vi "CC Create Script.vi"(11 "script name in":string) -> (3 "script name out":string)   [LabVIEW 2024]
uses:
  typedefs/CC cluster Exposure.ctl
  Detector/Detector Class/Detector enum Detector Integration Mode.ctl
  typedefs/CC cluster sidereal rate.ctl
  typedefs/CC Dithering.ctl
  typedefs/CC cluster Offset Dithering.ctl
  typedefs/CC Dithering Offsets.ctl
  typedefs/cc cluster muRA muDEC.ctl
  typedefs/CC cluster Random Dithering.ctl
  Detector/FITS/FITS enum Data Type.ctl
  Telescope/CC cluster Telescope Offsets.ctl
  typedefs/CC cluster Object.ctl
  typedefs/CC cluster RA and DEC.ctl
  typedefs/CC Script Step.ctl
  typedefs/CC enum Script Action.ctl
  Scripts/CC Rd Wr Script Creator Defaults.ctl
  typedefs/CC Dithering Map.ctl
  typedefs/CC enum Dithering Types.ctl
  Detector/FITS/FITS cluster Header Row.ctl
  typedefs/CC cluster Script.ctl
  Subsystems/SS typedef cluster Instrument Command Queue Data.ctl
  Scripts/CC Rd Wr Script Action.ctl
  Focus/Focus cluster MoveFocus Command Parameters.ctl
  typedefs/CC cluster Filter Wheel Parameters.ctl
  typedefs/CC cluster Acquire Parameters.ctl
  typedefs/CC cluster Pause Parameters.ctl
  Filter Wheel/Filter Wheel Object/Filter Wheel.lvclass
  Telescope/PRIME Telescope/PRIME Telescope.lvclass
panel:
  in  "Script Path":path
  in  "Delete":bool
  in  "New Button":bool
  in  "Save As Button":bool
  in  "Script Name":u16(ring) items=["SouthernCross"]
  in  "Save Script":bool
  in  "Close":bool
  in  "Script":i32(listbox)
  in  "Tab Control":T1(tab)
  in  "Units":string
  in  "Open Button":bool
  out "FITS Header Template":path
  in  "Save Header":bool
  in  "Add/Replace":bool
  in  "Comment":string
  in  "Value":string
  in  "Header Field":string(combo)
  in  "FITS Header":i32(listbox)
  in  "Type":T2
  in  "RA and DEC String":cluster{"RA":string, "DEC":string}={"RA"="HH:MM:SS.nnn", "DEC"="DEG:arcmin:arcsec.nn"} caption="RA and DEC"
  in  "Obj Add to Script":bool
  in  "Obj Remove":bool
  in  "Object Name":cluster{"Name":string}
  in  "Sidereal Rate":T3
  in  "Obj Add/Replace":bool
  in  "Objects":i32(listbox)
  in  "Proper Motion":T4
  in  "Offsets":T5
  in  "Exp Add to Script":bool
  in  "Exp Remove":bool
  in  "Exp Add/Replace":bool
  in  "Exposure":T6={"Mode"=enum."CDS", "Integration Time"=1.0, "Name"="", "Images"=1}
  in  "Exposures":i32(listbox)
  in  "Add FW 4":bool
  in  "Add FW 3":bool
  in  "Add FW 2":bool
  in  "Add FW 1":bool
  in  "Filter Wheel 4":i32(listbox)
  in  "Filter Wheel 3":i32(listbox)
  in  "Filter Wheel 2":i32(listbox) caption="OuterWheel"
  in  "Filter Wheel 1":i32(listbox) caption="InnerWheel"
  in  "Name":string
  in  "Dither Add to Script":bool
  in  "Dithering Add/Replace":bool
  in  "Dithering":i32(listbox)
  in  "Dithering Remove":bool
  in  "Dither Select":enum32{"Random", "Offset"}(tab)
  in  "Random Dither":T8={"Count"=1, "Radius"=1.0, "Name"=""}
  in  "Dithering Offset":T9
  in  "Add Image Acq":bool
  in  "Acquire Parameters":T12
  in  "Add Macro":bool
  in  "Script to Call":u16(ring)
  in  "Move Telescope":bool
  in  "RA and DEC String 2":cluster{"RA":string, "DEC":string}={"RA"="HH:MM:SS.nnn", "DEC"="DEG:arcmin:arcsec.nn"} caption="RA and DEC"
  in  "Telescope Focus":T13
  in  "Message for User":string
  in  "Add Ask":bool caption="Add Ask to Script"
  in  "Seconds to Pause":dbl=10.0
  in  "Add Pause":bool caption="Add Pause to Script"
  in  "Home":bool
  in  "Absolute":bool
  in  "Relative":bool
  in  "Steps":i32
  in  "Select Motor (0:n-1)":i32 min=0 max=3 step=1
  in  "Add No-op":bool caption="Add Noop to Script"
  out "Script As Text":string="DefineObject Alpha1234 Standard RA=123.456 DEC=456.789\nDefineExposure Number=1,Groups=1,ReadoutsPerGroup=1,TimeBetweenGroups=10,TimeBetweenReadouts=10\nDefineDithering DEC=0,-10,+10 RA=0,-10,+10\nMoveFilter A,B\nAcquireImages [This command acquires image at every dithering position]\n\n"
  in  "Send":bool
  in  "Script Line":string
  # "Select a Configuration (PRIME or RIMAS, FilterWheel, etc.)"
  # "Add warning for invalid combinationss"
  # "\"\t   Y, J, or H can go with Open or Narrow only\n\"\t  Z must go with Open\n\"\t Dark can go with anything\n\"\t Open can go with anything\n\"\t Narrow can only go with T, J, H"
  # "arcseconds"
  # "arcseconds"
  # "Telescope Pointing"
  # "Focus"
  # "The noop command is used for testing purposes. There are no parameters."
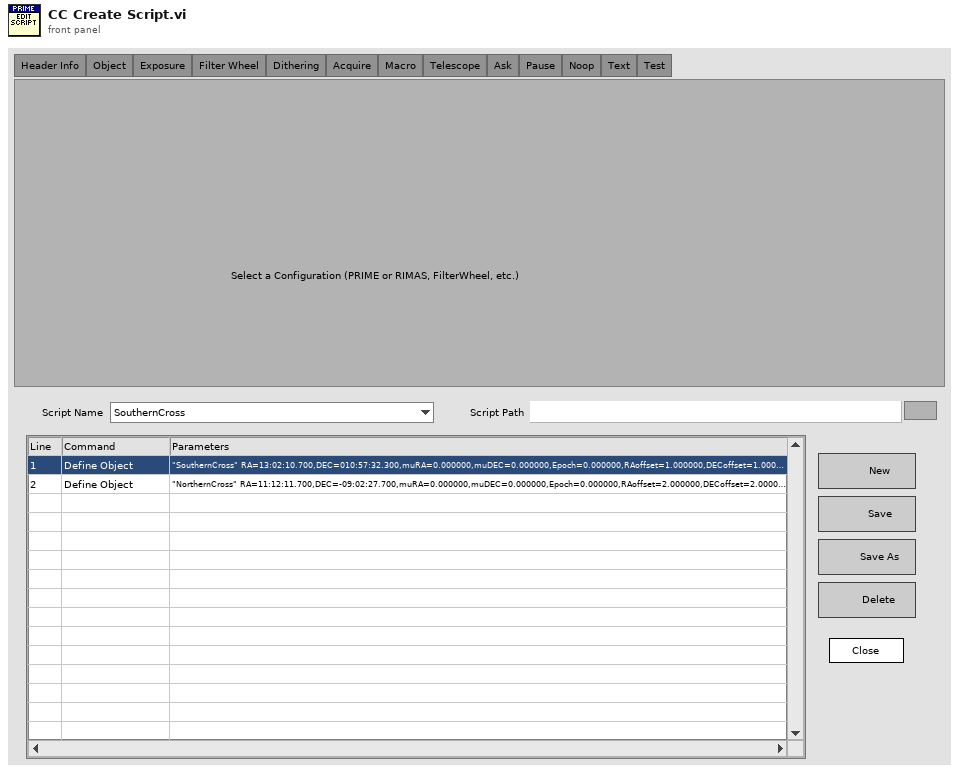
[diagram p1: front panel]
types:
  T1 = enum32{"Setup", "Header Info", "Object", "Exposure", "Filter Wheel", "Dithering", "Acquire", "Macro", "Telescope", "Ask", "Pause", "PicoMotors", "Noop", "Text", "Test"}
  T2 = typedef "FITS enum Data Type.ctl" = enum16{"String", "Integer", "Float"}
  T3 = typedef "CC cluster sidereal rate.ctl" = cluster{"dRA":dbl, "dDEC":dbl}
  T4 = typedef "cc cluster muRA muDEC.ctl" = cluster{"muRA":dbl, "muDEC":dbl, "Epoch":dbl}
  T5 = typedef "CC cluster Telescope Offsets.ctl" = cluster{"RA":dbl, "DEC":dbl, "ROT":dbl}
  T6 = typedef "CC cluster Exposure.ctl" = cluster{"Mode":T7, "Integration Time":dbl, "Name":string, "Images":i32}
  T7 = typedef "Detector enum Detector Integration Mode.ctl" = enum16{"SSR", "CDS", "MEAN", "MEDIAN", "MODE", "MIIN", "MAX"}
  T8 = typedef "CC cluster Random Dithering.ctl" = cluster{"Count":i32, "Radius":dbl, "Name":string}
  T9 = typedef "CC Dithering.ctl" = cluster{"Name":string, "Dithering Offsets":T10}
  T10 = typedef "CC cluster Offset Dithering.ctl" = cluster{"Offsets":T11[]}
  T11 = typedef "CC Dithering Offsets.ctl" = cluster{"DEC":dbl, "RA":dbl}
  T12 = cluster{"Object":string, "Exposure":string, "Dithering":string}
  T13 = cluster{"Focus Home":bool, "Move Focus":bool, "Position":dbl}
  T14 = typedef "CC cluster Object.ctl" = cluster{"Object":cluster{"Name":string}, "Sidereal Rate":T3, "RA and DEC":T15, "muRA muDEC Epoch":T4, "Offsets":T5}
  T15 = typedef "CC cluster RA and DEC.ctl" = cluster{"RA":dbl, "DEC":dbl}
  T16 = typedef "CC Script Step.ctl" = cluster{"Action":T17, "Data":variant}
  T17 = typedef "CC enum Script Action.ctl" = enum16{"Noop", "Define Object", "Define Exposure", "Define Dithering", "Acquire Images", "Set Filter Wheel", "Telescope Home", "Telescope Move", "Telescope RA DEC", "Focus Move Relative", "Focus Move Absolute", "Focus Set Home", "Macro", "Pause", "Ask User", "Define Random Dither"}
  T18 = typedef "CC Rd Wr Script Creator Defaults.ctl" = cluster{"Script":string, "Script Path":path}
  T19 = typedef "CC Dithering Map.ctl" = cluster{"Name":string, "Dithering Offsets":T9, "Dithering Type":T20, "Random Dither":T8}
  T20 = typedef "CC enum Dithering Types.ctl" = enum16{"Random", "Offsets", "None"}
  T21 = typedef "FITS cluster Header Row.ctl" = cluster{"Field Name":string, "Type":T2, "Value":string, "Comment":string, "Units":string}
  T22 = cluster{"state":refnum<user-event>, "Object Map":map{string, T14}, "curr object":string, "Exp Map":map{string, T6}, "Script":T16[], "Settings":T18, "test":T16[], "Dither Map":map{string, T19}, "Hdr Map":map{string, T21}}
  T23 = typedef "CC cluster Script.ctl" = cluster{"Name":string, "Script":T16[]}
  T24 = typedef "CC Rd Wr Script Action.ctl" = enum16{"Read", "Write", "List", "Delete"}
  T25 = typedef "SS typedef cluster Instrument Command Queue Data.ctl" = cluster{"Cmd":string, "Parameters":variant}
  T26 = typedef "Focus cluster MoveFocus Command Parameters.ctl" = cluster{"Motor":i32, "Position":i32}
  T27 = typedef "CC cluster Filter Wheel Parameters.ctl" = cluster{"Wheel":i32, "Filter":i32}
  T28 = enum32{"Setup", "Object", "Exposure", "Dithering", "Acquire", "Filter Wheel", "Focus", "Macro", "Ask", "Pause", "Noop", "Text", "Test"}
  T29 = enum32{"Setup", "Object", "Exposure", "Dithering", "Acquire", "Filter Wheel", "Focus", "Ask", "Pause", "Noop", "Text", "Test"}
  T30 = typedef "CC cluster Acquire Parameters.ctl" = cluster{"Object":string, "Exposure":string, "Dithering":string}
  T31 = enum32{"Setup", "Object", "Exposure", "Filter Wheel", "Dithering", "Acquire", "Macro", "Telescope", "Ask", "Pause", "PicoMotors", "Noop", "Text", "Test"}
  T32 = typedef "CC cluster Pause Parameters.ctl" = cluster{"Time (s)":dbl}
  T33 = typedef "CC cluster Script Panel Defaults.ctl" = cluster{"Script Name":string, "Script Path":path}
  T34 = typedef "RIMAS Detector Config.ctl" = cluster{"Detector":u16, "Offsets":u16[][], "Detector Computer":T35, "FITS hdr template0":path, "FITS hdr template1":path, "FITS Data File Path":path, "FITS Detector Settings":T36, "Sim Folder":path, "Integration Mode":T7, "Integration Time":dbl, "Frame Int Time":dbl}
  T35 = typedef "RIMAS Detector Server Config.ctl" = cluster{"Machine":string, "Password":string, "FITS File Path":string, "Port":u16, "Header Path":string, "Name":string}
  T36 = typedef "RIMAS Observation Config.ctl" = cluster{"Exp Time Short":dbl, "# of Frames":dbl, "Exp Time Long":dbl, "# of Groups":dbl, "Object Name":string, "Object":string, "Obs Type":string, "Image Type":string, "Observer":string, "Observer Affiliation":string}
  T37 = typedef "CC cluster Hardware Config.ctl" = cluster{"Installed Hardware":T38[]}
  T38 = typedef "CC cluster Device Index.ctl" = cluster{"Device Type Name":string, "Curr Device Name":string, "All Instances":string[]}
  T39 = typedef "Filter Wheel.lvclass/Filter Wheel configuration.ctl" = cluster{"Num Wheels":i32, "Filters":T40[], "Invalid Combinations":i32[][], "Addr":refnum<visa-resource-name>, "Name":string, "Simulate":bool, "Homing Parameters":T41, "Default Speed":u16}
  T40 = typedef "Filter Wheel.lvclass/Filter Wheel Details.ctl" = cluster{"Names":string[], "Relative Position":i32[], "Wheel Name":string}
  T41 = typedef "Filter Wheel Arduino Homing cluster.ctl" = cluster{"Direction (F: CW)":bool, "Speed":i32, "Accel":i32, "Min Distance":i32, "Short Leg":i32, "Error Cnts":i32}
  T42 = typedef "LVPoint32TypeDef.ctl" = cluster{"Horizontal":i32, "Vertical":i32}
  T43 = typedef "LVRowAndColumnTypeDef.ctl" = cluster{"Row":i32, "Column":i32}
  T44 = enum32{"Setup", "Object", "Exposure", "Dithering", "Acquire", "Filter Wheel", "Ask", "Pause", "Noop", "Text"}
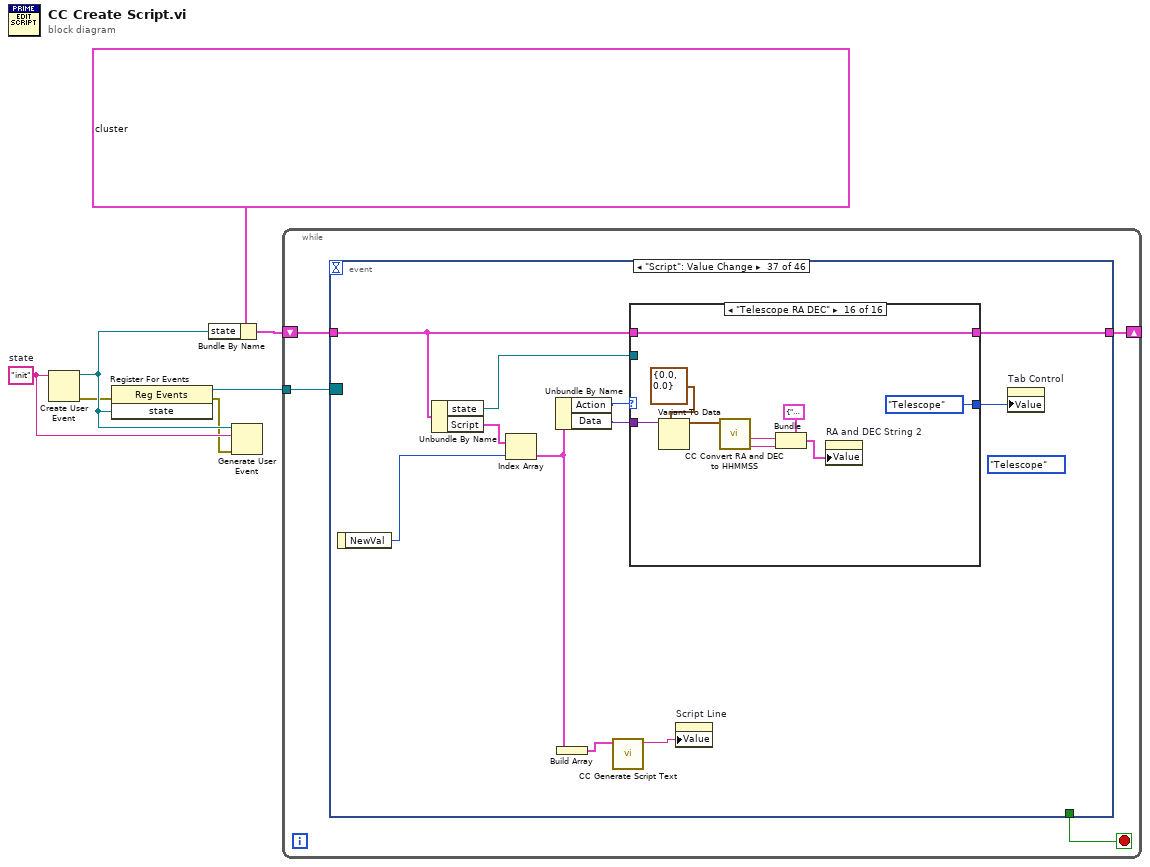
[diagram p0: block diagram]
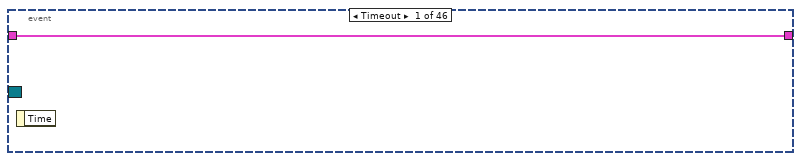
[diagram p2: hidden frame]
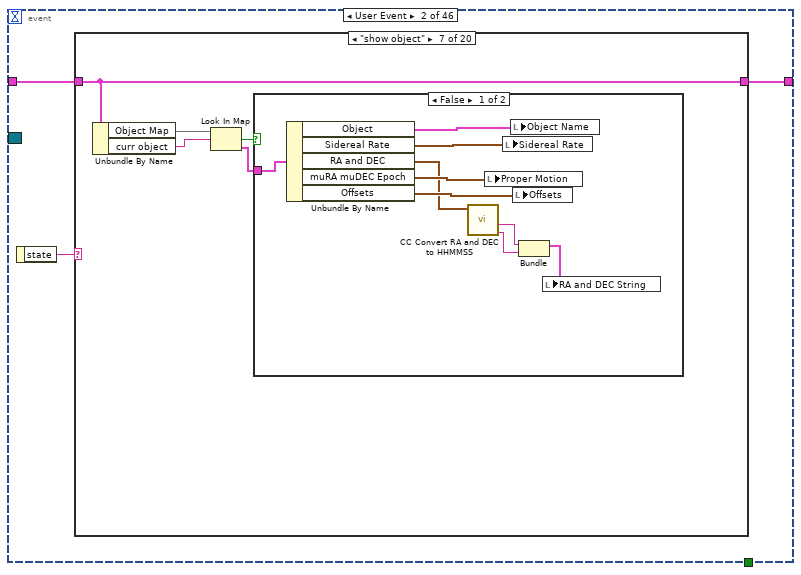
[diagram p3: hidden frame]
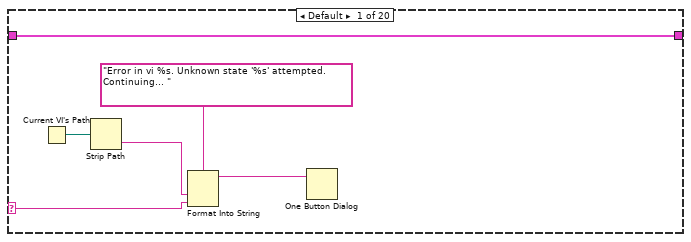
[diagram p4: hidden frame]
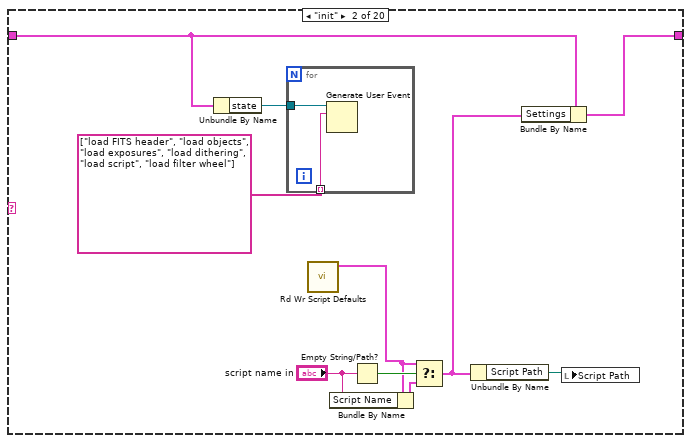
[diagram p5: hidden frame]
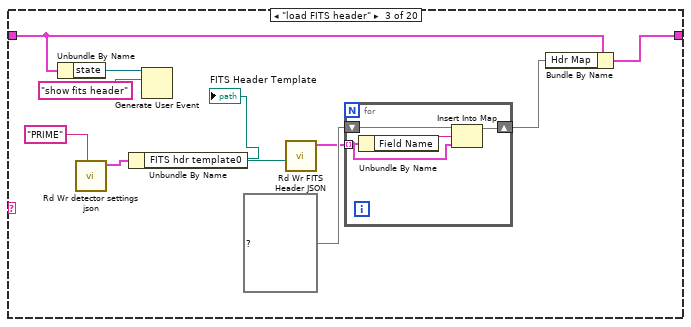
[diagram p6: hidden frame]
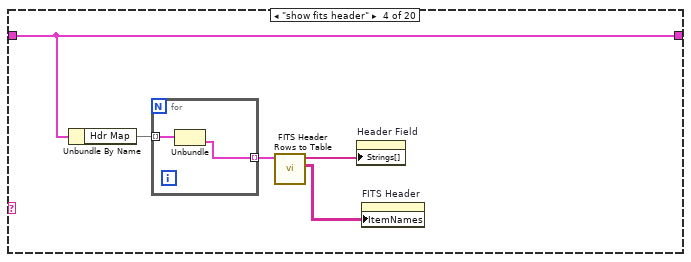
[diagram p7: hidden frame]
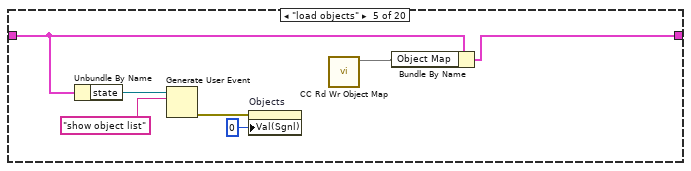
[diagram p8: hidden frame]
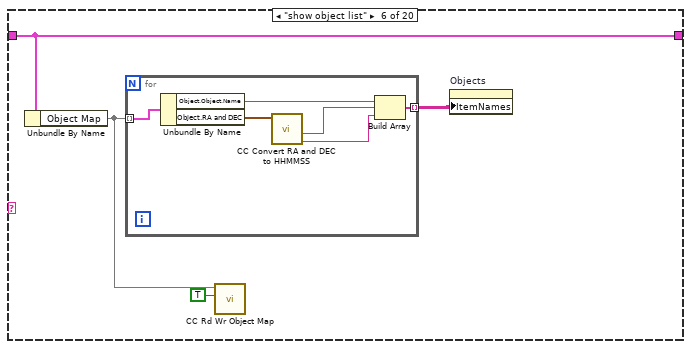
[diagram p9: hidden frame]
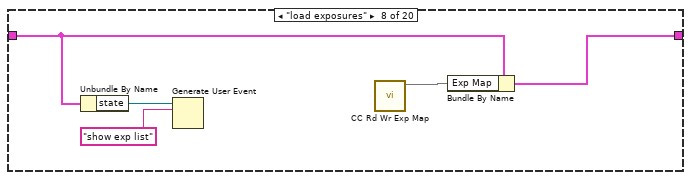
[diagram p11: hidden frame]
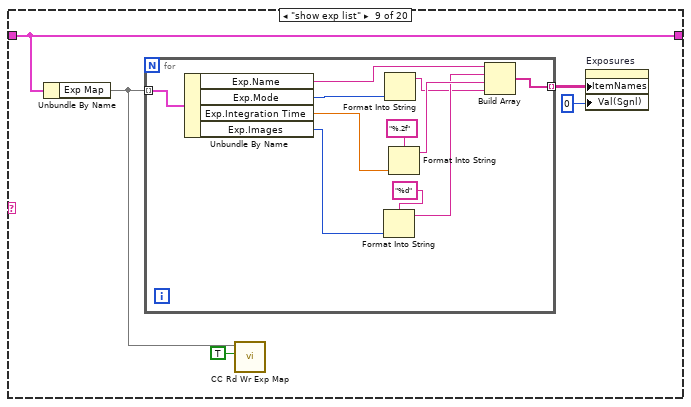
[diagram p12: hidden frame]
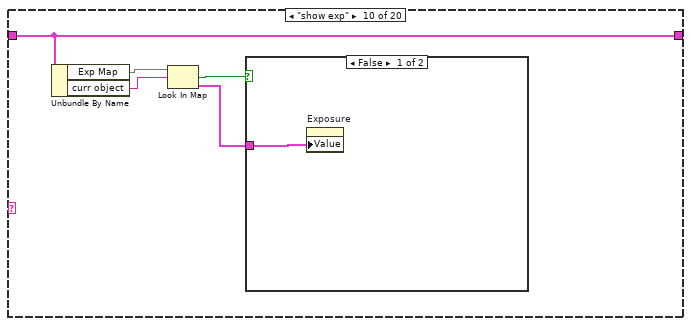
[diagram p13: hidden frame]
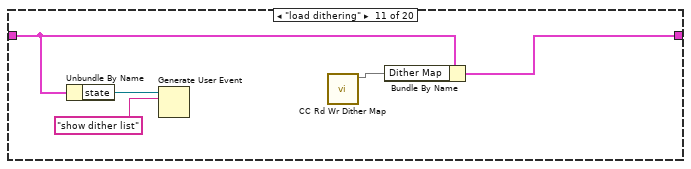
[diagram p15: hidden frame]
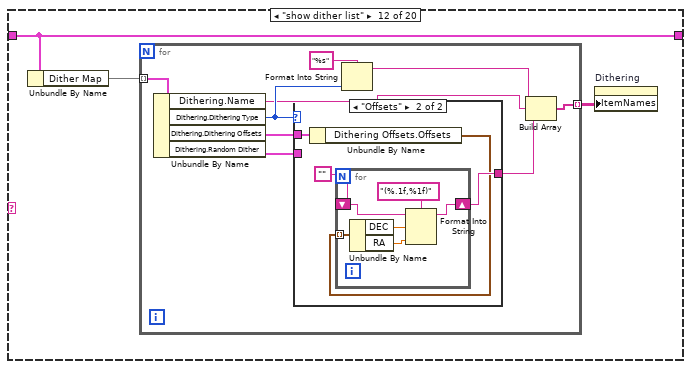
[diagram p16: hidden frame]
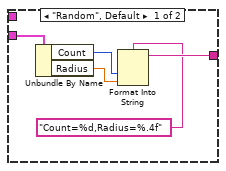
[diagram p17: hidden frame]
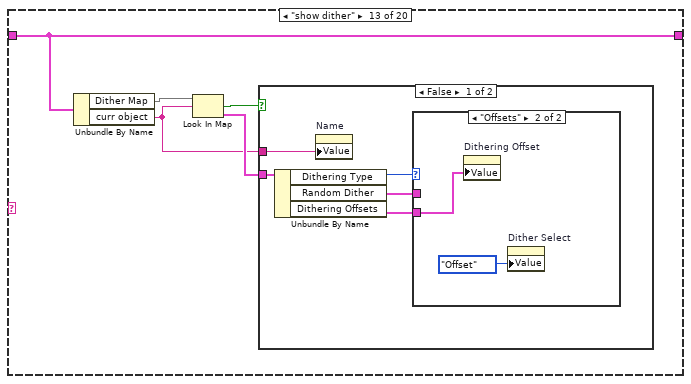
[diagram p18: hidden frame]
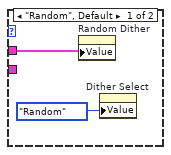
[diagram p19: hidden frame]
diagram:
  w3 = "init"  # state
  n1 = Create User Event(user event datatype=w3) -> (user event=w5:refnum<user-event>, error out=w1:errorcluster)  [unwired: 1 in]
  n2 = register-events(error in=w1, w5) -> (reference out=w4:refnum<event-registration>, error out=w2:errorcluster)  [unwired: 1 in]
  n3 = Bundle By Name(cluster=T22 {"state"=refnum, "Object Map"={}, "curr object"="", "Exp Map"={}, "Script"=[], "Settings"={"Script"="", "Script Path"=path ""}, "test"=[], "Dither Map"={}, "Hdr Map"={}}, "state"=w5) -> (w6:T22)
  n4 = Generate User Event(user event=w5, event data cluster=w3, error in=w2) -> ()  [unwired: 1 in, 2 out]
  n5 = while {
    tunnel: w4 -> [w11]
    shift-right: [w9] -> _
    shift-left: w6 -> [w10]
    stop <- w8 stop-if-true
    n6 = event shown="[36] \"Script\": Value Change" {
      selector: w11 -> [_ _ _ _ _ _ _ _ _ _ _ _ _ _ _ _ _ _ _ _ _ _ _ _ _ _ _ _ _ _ _ _ _ _ _ _ _ _ _ _ _ _ _ _ _ _]
      dyn-events: _ -> [_ _ _ _ _ _ _ _ _ _ _ _ _ _ _ _ _ _ _ _ _ _ _ _ _ _ _ _ _ _ _ _ _ _ _ _ _ _ _ _ _ _ _ _ _ _]
      timeout: _ -> [_ _ _ _ _ _ _ _ _ _ _ _ _ _ _ _ _ _ _ _ _ _ _ _ _ _ _ _ _ _ _ _ _ _ _ _ _ _ _ _ _ _ _ _ _ _]
      tunnel: w10 -> [w12 w14 w271 w283 w285 w288 w310 w324 w328 w339 w341 w352 w365 w386 w390 w402 w412 w432 w447 w470 w495 w526 w537 w543 w558 w572 w609 w615 w636 w675 w686 w698 w703 w714 w720 w728 w779 w886 w900 w913 w922 w934 w949 w951 w985 w989]
      tunnel: [w12 w13 w272 w283 w285 w289 w310 w324 w328 w336 w342 w353 w366 w387 w391 w403 w413 w433 w446 w469 w494 w527 w538 w544 w559 w573 w610 w614 w636 w676 w687 w698 w702 w714 w721 w728 w778 w887 w901 w914 w923 w935 w949 w950 w985 w989] -> w9
      tunnel: [_ _ _ _ _ _ _ _ _ _ _ _ _ _ _ _ _ _ _ _ _ _ _ _ _ _ _ _ _ _ _ _ _ _ _ _ _ _ _ _ _ _ _ _ _ "Close"] -> w8
      event Timeout {
        n7 = event-data() -> ()  [unwired: 1 in, 1 out]
      }
      event User Event {
        n8 = event-data() -> ("state"=w15:string)  [unwired: 1 in]
        n9 = case shown="\"show object\"" w15 {
          selector: w15 -> [w20 _ _ _ _ _ _ _ _ _ _ _ _ _ _ _ _ _ _ _]
          tunnel: w14 -> [w16 w28 w36 w50 w59 w64 w76 w86 w95 w111 w114 w120 w146 w163 w202 w230 w235 w250 w255 w258]
          tunnel: [w16 w29 w41 w50 w61 w64 w76 w89 w95 w111 w117 w120 w146 w164 w202 w230 w235 w250 w255 w258] -> w13
          frame Default {
            n10 = Current VI's Path() -> (path=w19:path)
            n11 = Strip Path(path=w19) -> (name=w18:string)  [unwired: 1 out]
            n12 = Format Into String(format string="Error in vi %s. Unknown state '%s' attempted. Continuing... ", w18, w20) -> (resulting string=w17:string)  [unwired: 2 in, 1 out]
            n13 = One Button Dialog(message=w17) -> ()  [unwired: 1 in, 1 out]
          }
          frame "init" {
            n14 = Unbundle By Name(w28) -> ("state"=w31:refnum<user-event>)
            n15 = for {
              tunnel: w31 -> [w33]
              tunnel: string[] ["load FITS header", "load objects", "load exposures", "load dithering", "load script", "load filter wheel"] -> [w32] mode=indexing
              n16 = Generate User Event(user event=w33, event data cluster=w32) -> ()  [unwired: 2 in, 2 out]
            }
            n17 = call "Rd Wr Script Defaults.vi"() -> ("Script Settings"=w22:T33)  [unwired: 10 in, 1 out]
            n18 = Bundle By Name(cluster=w22, "Script Name"="script name in") -> (w25:T33)
            n19 = Empty String/Path?(string/path="script name in") -> (empty?=w27:bool)
            n20 = Select(t=w22, s=w27, f=w25) -> (s? t:f=w23:T33)
            n21 = Unbundle By Name(w23) -> ("Script Path"=w24:path)
            n22 = Bundle By Name(cluster=w28, "Settings"=w23) -> (w29:T22)
            n23 = local write "Script Path"(w24) -> ()
          }
          frame "load FITS header" {
            n24 = Unbundle By Name(w36) -> ("state"=w35:refnum<user-event>)
            n25 = call "Rd Wr detector settings json.vi"("Detector Name"="PRIME") -> ("Detector Config"=w42:T34)  [unwired: 9 in, 1 out]
            n26 = Unbundle By Name(w42) -> ("FITS hdr template0"=w40:path)
            "FITS Header Template" <- w40
            n27 = Generate User Event(user event=w35, event data cluster="show fits header" ("event data")) -> ()  [unwired: 2 in, 2 out]
            n28 = call "Rd Wr FITS Header JSON.vi"("FITS Template"=w40) -> ("FITS Hdr Rows"=w37:T21[])  [unwired: 9 in, 1 out]
            n29 = for {
              tunnel: w37 -> [w45] mode=indexing
              shift-right: [w44] -> w38
              shift-left: map{string, T21} {} ("Hdr Map") -> [w47]
              n30 = Unbundle By Name(w45) -> ("Field Name"=w46:string)
              n31 = Insert Into Map(map in=w47, key=w46, value=w45) -> (map out=w44:map{string, T21})  [unwired: 2 out]
            }
            n32 = Bundle By Name(cluster=w36, "Hdr Map"=w38) -> (w41:T22)
          }
          frame "show fits header" {
            n33 = Unbundle By Name(w50) -> ("Hdr Map"=w49:map{string, T21})
            n34 = for {
              tunnel: w49 -> [w54] mode=indexing
              tunnel: [w53] -> w48 mode=indexing
              n35 = Unbundle(w54) -> (w53:T21)  [unwired: 1 out]
            }
            n36 = call "FITS Header Rows to Table.vi"("FITS Hdr Rows"=w48) -> ("table"=w51:string[][], "Keywords"=w52:string[])  [unwired: 9 in]
            n37 = property on="Header Field" class="CmbBox"("Strings[]"=w52) -> ()  [unwired: 2 in, 2 out]
            n38 = property on="FITS Header" class="MCListbox (strict)"("ItemNames"=w51) -> ()  [unwired: 2 in, 2 out]
          }
          frame "load objects" {
            n39 = Unbundle By Name(w59) -> ("state"=w58:refnum<user-event>)
            n40 = Generate User Event(user event=w58, event data cluster="show object list" ("event data")) -> (error out=w56:errorcluster)  [unwired: 2 in, 1 out]
            n41 = property on="Objects" class="MCListbox (strict)"(error in=w56, "Val(Sgnl)"=0 ("Value (Signaling)")) -> ()  [unwired: 1 in, 2 out]
            n42 = call "CC Rd Wr Object Map.vi"() -> ("Object Map in"=w60:map{string, T14})  [unwired: 10 in, 1 out]
            n43 = Bundle By Name(cluster=w59, "Object Map"=w60) -> (w61:T22)
          }
          frame "show object list" {
            n44 = Unbundle By Name(w64) -> ("Object Map"=w63:map{string, T14})
            n45 = for {
              tunnel: w63 -> [w71] mode=indexing
              tunnel: [w69] -> w65 mode=indexing
              n46 = Unbundle By Name(w71) -> ("Object.Object.Name"=w70:string, "Object.RA and DEC"=w68:T15)
              n47 = call "CC Convert RA and DEC to HHMMSS.vi"("RA and DEC"=w68) -> ("DEC String"=w66:string, "RA String"=w67:string)  [unwired: 9 in]
              n48 = Build Array(w70, w67, w66) -> (w69:string[])
            }
            n49 = call "CC Rd Wr Object Map.vi"("Write? (F:Read)"=TRUE, "Object Map in"=w63) -> ()  [unwired: 8 in, 2 out]
            n50 = property on="Objects" class="MCListbox (strict)"("ItemNames"=w65) -> ()  [unwired: 2 in, 2 out]
          }
          frame "show object" {
            n51 = Unbundle By Name(w76) -> ("Object Map"=w75:map{string, T14}, "curr object"=w74:string)
            n52 = Look In Map(map=w75, key=w74) -> (key not found?=w73:bool, value=w72:T14)  [unwired: 1 in]
            n53 = case shown="False" w73 {
              tunnel: w72 -> [w85 _]
              frame False {
                n54 = Unbundle By Name(w85) -> ("Object"=w84:cluster{"Name":string}, "Sidereal Rate"=w83:T3, "RA and DEC"=w80:T15, "muRA muDEC Epoch"=w82:T4, "Offsets"=w81:T5)
                n55 = call "CC Convert RA and DEC to HHMMSS.vi"("RA and DEC"=w80) -> ("DEC String"=w78:string, "RA String"=w79:string)  [unwired: 9 in]
                n56 = local write "Proper Motion"(w82) -> ()
                n57 = local write "Sidereal Rate"(w83) -> ()
                n58 = local write "Object Name"(w84) -> ()
                n59 = local write "Offsets"(w81) -> ()
                n60 = Bundle("RA String"=w79, "DEC String"=w78) -> (w77:cluster{"RA String":string, "DEC String":string})  [unwired: 1 in]
                n61 = local write "RA and DEC String"(w77) -> ()
              }
              frame True {
              }
            }
          }
          frame "load exposures" {
            n62 = Unbundle By Name(w86) -> ("state"=w88:refnum<user-event>)
            n63 = Generate User Event(user event=w88, event data cluster="show exp list" ("event data")) -> ()  [unwired: 2 in, 2 out]
            n64 = call "CC Rd Wr Exp Map.vi"() -> ("Exp Map"=w90:map{string, T6})  [unwired: 10 in, 1 out]
            n65 = Bundle By Name(cluster=w86, "Exp Map"=w90) -> (w89:T22)
          }
          frame "show exp list" {
            n66 = Unbundle By Name(w95) -> ("Exp Map"=w93:map{string, T6})
            n67 = for {
              tunnel: w93 -> [w106] mode=indexing
              tunnel: [w102] -> w94 mode=indexing
              n68 = Unbundle By Name(w106) -> ("Exp.Name"=w105:string, "Exp.Mode"=w104:T7, "Exp.Integration Time"=w101:dbl, "Exp.Images"=w99:i32)
              n69 = Format Into String(format string="%d", w99) -> (resulting string=w97:string)  [unwired: 2 in, 1 out]
              n70 = Format Into String(w104) -> (resulting string=w96:string)  [unwired: 3 in, 1 out]
              n71 = Format Into String(format string="%.2f", w101) -> (resulting string=w100:string)  [unwired: 2 in, 1 out]
              n72 = Build Array(w105, w97, w100, w96) -> (w102:string[])
            }
            n73 = call "CC Rd Wr Exp Map.vi"("Write? (F:Read)"=TRUE, "Exp Map"=w93) -> ()  [unwired: 8 in, 2 out]
            n74 = property on="Exposures" class="MCListbox (strict)"("ItemNames"=w94, "Val(Sgnl)"=0 ("Value (Signaling)")) -> ()  [unwired: 2 in, 2 out]
          }
          frame "show exp" {
            n75 = Unbundle By Name(w111) -> ("Exp Map"=w110:map{string, T6}, "curr object"=w109:string)
            n76 = Look In Map(map=w110, key=w109) -> (key not found?=w108:bool, value=w107:T6)  [unwired: 1 in]
            n77 = case shown="False" w108 {
              tunnel: w107 -> [w112 _]
              frame False {
                n78 = property on="Exposure" class="Clust (strict)"("Value"=w112) -> ()  [unwired: 2 in, 2 out]
              }
              frame True {
              }
            }
          }
          frame "load dithering" {
            n79 = Unbundle By Name(w114) -> ("state"=w116:refnum<user-event>)
            n80 = Generate User Event(user event=w116, event data cluster="show dither list" ("event data")) -> ()  [unwired: 2 in, 2 out]
            n81 = call "CC Rd Wr Dither Map.vi"() -> ("Dither Map"=w113:map{string, T19})  [unwired: 10 in, 1 out]
            n82 = Bundle By Name(cluster=w114, "Dither Map"=w113) -> (w117:T22)
          }
          frame "show dither list" {
            n83 = Unbundle By Name(w120) -> ("Dither Map"=w118:map{string, T19})
            n84 = for {
              tunnel: w118 -> [w129] mode=indexing
              tunnel: [w126] -> w119 mode=indexing
              n85 = Unbundle By Name(w129) -> ("Dithering.Name"=w121:string, "Dithering.Dithering Type"=w123:T20, "Dithering.Dithering Offsets"=w128:T9, "Dithering.Random Dither"=w122:T8)
              n86 = case shown="\"Offsets\"" w123 {
                tunnel: w128 -> [_ w136]
                tunnel: [w131 w137] -> w127
                tunnel: w122 -> [w134 _]
                frame "Random", Default {
                  n87 = Unbundle By Name(w134) -> ("Count"=w133:i32, "Radius"=w132:dbl)
                  n88 = Format Into String(format string="Count=%d,Radius=%.4f", w133, w132) -> (resulting string=w131:string)  [unwired: 2 in, 1 out]
                }
                frame "Offsets" {
                  n89 = Unbundle By Name(w136) -> ("Dithering Offsets.Offsets"=w135:T11[])
                  n90 = for {
                    tunnel: w135 -> [w143] mode=indexing
                    shift-right: [w139] -> w137
                    shift-left: "" -> [w140]
                    n91 = Unbundle By Name(w143) -> ("DEC"=w142:dbl, "RA"=w141:dbl)
                    n92 = Format Into String(format string="(%.1f,%1f)", initial string=w140, w142, w141) -> (resulting string=w139:string)  [unwired: 1 in, 1 out]
                  }
                }
              }
              n93 = Format Into String(format string="%s", w123) -> (resulting string=w124:string)  [unwired: 2 in, 1 out]
              n94 = Build Array(w124, w121, w127) -> (w126:string[])
            }
            n95 = property on="Dithering" class="MCListbox (strict)"("ItemNames"=w119) -> ()  [unwired: 2 in, 2 out]
          }
          frame "show dither" {
            n96 = Unbundle By Name(w146) -> ("Dither Map"=w149:map{string, T19}, "curr object"=w145:string)
            n97 = Look In Map(map=w149, key=w145) -> (key not found?=w148:bool, value=w147:T19)  [unwired: 1 in]
            n98 = case shown="False" w148 {
              tunnel: w147 -> [w154 _]
              tunnel: w145 -> [w150 _]
              frame False {
                n99 = Unbundle By Name(w154) -> ("Dithering Type"=w153:T20, "Random Dither"=w151:T8, "Dithering Offsets"=w152:T9)
                n100 = property on="Name" class="Str"("Value"=w150) -> ()  [unwired: 2 in, 2 out]
                n101 = case shown="\"Offsets\"" w153 {
                  tunnel: w152 -> [_ w158]
                  tunnel: w151 -> [w156 _]
                  frame "Random", Default {
                    n102 = property on="Random Dither" class="Clust (strict)"("Value"=w156) -> ()  [unwired: 2 in, 2 out]
                    n103 = property on="Dither Select" class="TabCtl (strict)"("Value"=enum32{"Random", "Offset"}."Random" ("Dither Select")) -> ()  [unwired: 2 in, 2 out]
                  }
                  frame "Offsets" {
                    n104 = property on="Dithering Offset" class="Clust (strict)"("Value"=w158) -> ()  [unwired: 2 in, 2 out]
                    n105 = property on="Dither Select" class="TabCtl (strict)"("Value"=enum32{"Random", "Offset"}."Offset" ("Dither Select")) -> ()  [unwired: 2 in, 2 out]
                  }
                }
              }
              frame True {
              }
            }
          }
          frame "load script" {
            n106 = Unbundle By Name(w163) -> ("Settings.Script"=w161:string, "Settings.Script Path"=w159:path, "state"=w162:refnum<user-event>)
            n107 = Empty String/Path?(string/path=w161) -> (empty?=w160:bool)
            n108 = case shown="True" w160 {
              tunnel: [w175 w182] -> w164
              tunnel: w163 -> [w174 w182]
              tunnel: w162 -> [w173 _]
              tunnel: w161 -> [w169 _]
              tunnel: w159 -> [w165 _]
              frame False {
                n109 = Bundle By Name(cluster=T23 {"Name"="", "Script"=[]} ("Script"), "Name"=w169) -> (w178:T23)
                n110 = Generate User Event(user event=w173, event data cluster="show script" ("event data")) -> ()  [unwired: 2 in, 2 out]
                n111 = call "CC Rd Wr Script.vi"("Script Path"=w165, "Script"=w178) -> ("Syntax Errors"=w170:string, "Script List"=w168:string[], "Script"=w177:T23, "Script Ok?"=w171:bool)  [unwired: 4 in, 2 out]
                n112 = Unbundle By Name(w177) -> ("Script"=w176:T16[])
                n113 = Search 1D Array(1D array=w168, element=w169) -> (index of element=w167:i32)  [unwired: 1 in]
                n114 = case shown="False" w171 {
                  tunnel: w170 -> [w180 _]
                  frame False {
                    n115 = One Button Dialog(message=w180) -> ()  [unwired: 1 in, 1 out]
                  }
                  frame True {
                  }
                }
                n116 = property on="Script Name" class="Ring (strict)"("Strings []"=w168, "Value"=w167) -> ()  [unwired: 2 in, 2 out]
                n117 = Bundle By Name(cluster=w174, "Script"=w176) -> (w175:T22)
                n118 = Delete From Array(array=w168, index=w167) -> (array with subset deleted=w166:string[])  [unwired: 1 in, 1 out]
                n119 = property on="Script to Call" class="Ring (strict)"("Strings []"=w166) -> ()  [unwired: 2 in, 2 out]
              }
              frame True {
                n120 = property on="Script" class="MCListbox (strict)"("ItemNames"=string[][] [] ("Item Names")) -> ()  [unwired: 2 in, 2 out]
              }
            }
          }
          frame "load filter wheel" {
            n121 = call "CC Rd Wr Hardware Configuration.vi"() -> ("Hardware Config out"=w185:T37)  [unwired: 9 in, 2 out]
            n122 = control-ref of="Filter Wheel 4"() -> (w197:refnum<vi>)
            n123 = control-ref of="Add FW 1"() -> (w192:refnum<vi>)
            n124 = control-ref of="Add FW 2"() -> (w189:refnum<vi>)
            n125 = control-ref of="Add FW 3"() -> (w190:refnum<vi>)
            n126 = control-ref of="Add FW 4"() -> (w191:refnum<vi>)
            n127 = control-ref of="Filter Wheel 3"() -> (w198:refnum<vi>)
            n128 = control-ref of="Filter Wheel 2"() -> (w199:refnum<vi>)
            n129 = control-ref of="Filter Wheel 1"() -> (w200:refnum<vi>)
            n130 = Unbundle By Name(w185) -> ("Installed Hardware"=w184:T38[])
            n131 = Build Array(w192, w189, w190, w191) -> (w188:refnum<vi>[])
            n132 = Build Array(w200, w199, w198, w197) -> (w193:refnum<vi>[])
            n133 = call "CC Get Current Device.vi"("Device Type Name"="filter wheel", "Hardware.Installed Hardware"=w184) -> ("Curr Device Name"=w183:string)  [unwired: 7 in, 2 out]
            n134 = for {
              tunnel: [w208] -> w194 mode=indexing
              tunnel: w193 -> [w207] mode=indexing
              tunnel: w188 -> [w205] mode=indexing
              tunnel: [w203] -> w187 mode=indexing
              n135 = property class="LstBox (strict)"(reference=w207, "Visible"=FALSE) -> (reference out=w208:refnum<vi>)  [unwired: 1 in, 1 out]
              n136 = property class="Bool"(reference=w205, "Visible"=FALSE) -> (reference out=w203:refnum<vi>)  [unwired: 1 in, 1 out]
            }
            n137 = call "Rd Wr Filter Wheel Settings.vi"("Wheel Name"=w183) -> ("Filter Wheel Settings"=w201:T39)  [unwired: 9 in, 1 out]
            n138 = Unbundle By Name(w201) -> ("Filters"=w195:T40[])  [unwired: 1 out]
            n139 = for {
              N: 4 -> [_]
              tunnel: w195 -> [w214] mode=indexing
              tunnel: w194 -> [w213] mode=indexing
              tunnel: w187 -> [w211] mode=indexing
              w210 = TRUE ("Visible")
              n140 = Unbundle By Name(w214) -> ("Names"=w212:string[], "Wheel Name"=w209:string)
              n141 = property class="LstBox (strict)"(reference=w213, "Item Names"=w212, "Visible"=w210, "Caption.Text"=w209) -> ()  [unwired: 1 in, 2 out]
              n142 = property class="Bool"(reference=w211, "Visible"=w210) -> ()  [unwired: 1 in, 2 out]
            }
          }
          frame "save script" {
            n143 = Unbundle By Name(w230) -> ("Settings.Script"=w218:string, "Script"=w231:T16[], "Settings.Script Path"=w215:path)
            n144 = Bundle By Name(cluster=T23 {"Name"="", "Script"=[]} ("Script"), "Name"=w218, "Script"=w231) -> (w232:T23)
            n145 = Obtain Queue(name (unnamed)="Script Queue", element data type=T25 {"Cmd"="", "Parameters"=variant}) -> (queue out=w227:refnum<queue>)  [unwired: 3 in, 2 out]
            n146 = call "CC Rd Wr Script.vi"("Script Path"=w215, "Action"=CC_Rd_Wr_Script_Action."Write", "Script"=w232) -> ("error out"=w220:errorcluster, "Script List"=w219:string[])  [unwired: 3 in, 4 out]
            n147 = Bundle By Name(cluster=T25 {"Cmd"="", "Parameters"=variant} ("element"), "Cmd"="set script", "Parameters"=w218) -> (w223:T25)
            n148 = Search 1D Array(1D array=w219, element=w218) -> (index of element=w217:i32)  [unwired: 1 in]
            n149 = property on="Script Name" class="Ring (strict)"(error in=w220, "Strings []"=w219, "Value"=w217) -> (error out=w224:errorcluster)  [unwired: 1 in, 1 out]
            n150 = Enqueue Element(queue=w227, element=w223, error in (no error)=w224) -> (queue out=w221:refnum<queue>, error out=w222:errorcluster)  [unwired: 1 in, 1 out]
            n151 = Release Queue(queue=w221, error in (no error)=w222) -> ()  [unwired: 1 in, 3 out]
          }
          frame "delete script" {
            n152 = Unbundle By Name(w235) -> ("Settings.Script Path"=w234:path)
            n153 = property on="Script Name" class="Ring (strict)"() -> ("Strings []"=w243:string[], "Value"=w240:u16)  [unwired: 2 in, 2 out]
            n154 = Index Array(array=w243, index=w240) -> (element=w241:string)
            n155 = Bundle By Name(cluster=T23 {"Name"="", "Script"=[]} ("Script"), "Name"=w241) -> (w245:T23)
            n156 = call "CC Rd Wr Script.vi"("Script Path"=w234, "Action"=CC_Rd_Wr_Script_Action."Delete", "Script"=w245) -> ("error out"=w244:errorcluster, "Script List"=w237:string[])  [unwired: 3 in, 4 out]
            n157 = Array Size(array=w237) -> (size(s)=w236:i32)
            n158 = In Range and Coerce(upper limit=w236, x=w240, lower limit=u16 0) -> (coerced(x)=w238:i32)  [unwired: 1 out]
            n159 = property on="Script Name" class="Ring (strict)"(error in=w244, "Strings []"=w237, "Val(Sgnl)"=w238) -> ()  [unwired: 1 in, 2 out]
          }
          frame "show script" {
            n160 = Unbundle By Name(w250) -> ("Script"=w249:T16[])
            n161 = call "CC Script to Table.vi"("Line Numbers?"=TRUE, "Script"=w249) -> ("table"=w248:string[][])  [unwired: 8 in, 1 out]
            n162 = property on="Script" class="MCListbox (strict)"("ItemNames"=w248) -> ()  [unwired: 2 in, 2 out]
          }
          frame "update script" {
            n163 = Unbundle By Name(w255) -> ("state"=w254:refnum<user-event>)
            n164 = Generate User Event(user event=w254, event data cluster="show script" ("event data")) -> (user event out=w253:refnum<user-event>)  [unwired: 2 in, 1 out]
            n165 = Generate User Event(user event=w253, event data cluster="save script" ("event data")) -> ()  [unwired: 2 in, 2 out]
          }
          frame "run test" {
            n166 = Unbundle By Name(w258) -> ("test"=w257:T16[])
            n167 = Index Array(array=w257) -> (element=w256:T16)  [unwired: 1 in]
            n168 = call "CC Script Execute Step.vi"("Script Step"=w256) -> ()  [unwired: 10 in, 1 out]
          }
        }
      }
      event "Add/Replace": Value Change {
        n169 = event-data() -> ()  [unwired: 1 in, 1 out]
        n170 = case shown="\"Integer\"" "Type" {
          tunnel: "Value" -> [w273 w276 w279]
          tunnel: [w273 w274 w277] -> w260
          frame "String", Default {
          }
          frame "Integer" {
            n171 = Decimal String To Number(string=w276) -> (number=w275:i32)  [unwired: 2 in, 1 out]
            n172 = Number To Decimal String(number=w275) -> (decimal integer string=w274:string)  [unwired: 1 in]
          }
          frame "Float" {
            n173 = Fract/Exp String To Number(string=w279) -> (number=w278:dbl)  [unwired: 3 in, 1 out]
            n174 = Number To Fractional String(number=w278) -> (F-format string=w277:string)  [unwired: 3 in]
          }
        }
        n175 = Unbundle By Name(w271) -> ("state"=w264:refnum<user-event>, "Hdr Map"=w267:map{string, T21})
        n176 = Bundle By Name(cluster=T21 {"Field Name"="", "Type"=enum."String", "Value"="", "Comment"="", "Units"=""} ("FITS Hdr Row"), "Field Name"="Header Field", "Type"="Type", "Value"=w260, "Comment"="Comment", "Units"="Units") -> (w266:T21)
        n177 = Insert Into Map(map in=w267, key="Header Field", value=w266) -> (map out=w265:map{string, T21})  [unwired: 2 out]
        n178 = Generate User Event(user event=w264, event data cluster="show fits header" ("event data")) -> ()  [unwired: 2 in, 2 out]
        n179 = Bundle By Name(cluster=w271, "Hdr Map"=w265) -> (w272:T22)
      }
      event "Header Field": Value Change {
        n180 = event-data() -> ("CtlRef"=w282:refnum<vi>, "NewVal"=w281:string)  [unwired: 1 in]
        n181 = call "FITS Filter Name.vi"("Hdr Name"=w281) -> ("Filtered Name"=w280:string)  [unwired: 9 in, 1 out]
        n182 = property class="CmbBox"(reference=w282, "Value"=w280) -> ()  [unwired: 1 in, 2 out]
      }
      event "FITS Header": Shortcut Menu Activation? {
        n183 = event-data() -> ()  [unwired: 1 in, 7 out]
        n184 = event-data("Discard?"=FALSE) -> ()  [unwired: 1 in, 1 out]
      }
      event "FITS Header": Shortcut Menu Selection (User) {
        n185 = event-data() -> ("ItemTag"=w294:string, "CtlRef"=w296:refnum<vi>, "Coords"=w295:T42)  [unwired: 1 in, 5 out]
        n186 = Unbundle By Name(w288) -> ("state"=w287:refnum<user-event>, "Hdr Map"=w291:map{string, T21})
        n187 = invoke class="MCListbox (strict)" method="Point To Row Column"(reference=w296, "Point"=w295) -> (reference out=w292:refnum<vi>, "CellPosition"=w293:T43)  [unwired: 5 in, 5 out]
        n188 = Generate User Event(user event=w287, event data cluster="show fits header" ("event data")) -> ()  [unwired: 2 in, 2 out]
        n189 = case shown="\"False\", Default" w294 {
          tunnel: w293 -> [_ w305]
          tunnel: w292 -> [_ w304]
          tunnel: w291 -> [w297 w300]
          tunnel: [w297 w298] -> w290
          frame "False", Default {
          }
          frame "Delete Item" {
            n190 = property class="MCListbox (strict)"(reference=w304) -> ("ItemNames"=w303:string[][])  [unwired: 1 in, 2 out]
            n191 = Unbundle By Name(w305) -> ("Row"=w302:i32)
            n192 = Index Array(array=w303, index (row)=w302, index (col)=0 ("disabled index (col)")) -> (element=w299:string)
            n193 = Remove From Map(10:w299, 11:w300) -> (3:w298:map{string, T21})  [unwired: 2 out]
          }
        }
        n194 = Bundle By Name(cluster=w288, "Hdr Map"=w290) -> (w289:T22)
      }
      event "FITS Header": Value Change {
        n195 = event-data() -> ("CtlRef"=w314:refnum<vi>, "NewVal"=w312:i32)  [unwired: 1 in]
        n196 = property class="MCListbox (strict)"(reference=w314) -> ("ItemNames"=w313:string[][])  [unwired: 1 in, 2 out]
        n197 = Unbundle By Name(w310) -> ("Hdr Map"=w309:map{string, T21})
        n198 = Index Array(array=w313, index (row)=w312, index (col)=0 ("disabled index (col)")) -> (element=w308:string)
        n199 = Look In Map(map=w309, key=w308) -> (key not found?=w307:bool, value=w306:T21)  [unwired: 1 in]
        n200 = case shown="False" w307 {
          tunnel: w306 -> [w320 _]
          frame False {
            n201 = Unbundle By Name(w320) -> ("Field Name"=w319:string, "Type"=w318:T2, "Value"=w317:string, "Comment"=w316:string, "Units"=w315:string)
            n202 = property on="Header Field" class="CmbBox"("Value"=w319) -> ()  [unwired: 2 in, 2 out]
            n203 = property on="Type" class="Enum (strict)"("Value"=w318) -> ()  [unwired: 2 in, 2 out]
            n204 = property on="Value" class="Str"("Value"=w317) -> ()  [unwired: 2 in, 2 out]
            n205 = property on="Units" class="Str"("Value"=w315) -> ()  [unwired: 2 in, 2 out]
            n206 = property on="Comment" class="Str"("Value"=w316) -> ()  [unwired: 2 in, 2 out]
          }
          frame True {
          }
        }
      }
      event "Open Button": Value Change {
        n207 = event-data() -> ()  [unwired: 1 in, 6 out]
        n208 = call "Rd Wr detector settings json.vi"("Detector Name"="PRIME") -> ("Detector Config"=w322:T34)  [unwired: 9 in, 1 out]
        n209 = Unbundle By Name(w322) -> ("FITS hdr template0"=w321:path)
        n210 = call <vilib>:"Show in File System.vi"("file or directory path"=w321) -> ()  [unwired: 10 in, 1 out]
      }
      event "Save Header": Value Change {
        n211 = event-data() -> ()  [unwired: 1 in, 6 out]
        n212 = call "Rd Wr detector settings json.vi"("Detector Name"="PRIME") -> ("Detector Config"=w330:T34)  [unwired: 9 in, 1 out]
        n213 = Unbundle By Name(w328) -> ("Hdr Map"=w327:map{string, T21})
        n214 = Unbundle By Name(w330) -> ("FITS hdr template0"=w329:path)
        n215 = for {
          tunnel: w327 -> [w333] mode=indexing
          tunnel: [w332] -> w326 mode=indexing
          n216 = Unbundle(w333) -> (w332:T21)  [unwired: 1 out]
        }
        n217 = call "Rd Wr FITS Header JSON.vi"("FITS Template"=w329, "Write? (F:Read)"=TRUE, "FITS Hdr Rows"=w326) -> ()  [unwired: 7 in, 2 out]
      }
      event "Script Path": Value Change {
        n218 = event-data() -> ()  [unwired: 1 in, 6 out]
        n219 = Unbundle By Name(w339) -> ("state"=w338:refnum<user-event>)
        n220 = Generate User Event(user event=w338, event data cluster="init" ("event data")) -> ()  [unwired: 2 in, 2 out]
        n221 = Bundle By Name(cluster=w339, "Settings.Script Path"="Script Path") -> (w336:T22)
        n222 = Unbundle By Name(w336) -> ("Settings"=w335:T18)
        n223 = call "Rd Wr Script Defaults.vi"("Write? (F:Read)"=TRUE, "Script Settings"=w335) -> ()  [unwired: 8 in, 2 out]
      }
      event "Telescope Focus.Focus Home": Value Change {
        n224 = event-data() -> ()  [unwired: 1 in, 6 out]
        n225 = Unbundle By Name(w341) -> ("Script"=w347:T16[], "state"=w344:refnum<user-event>)
        n226 = Generate User Event(user event=w344, event data cluster="update script" ("event data")) -> ()  [unwired: 2 in, 2 out]
        n227 = Bundle By Name(cluster=T16 {"Action"=enum."Acquire Images", "Data"=variant}, "Action"=CC_enum_Script_Action."Telescope Home") -> (w346:T16)
        n228 = Build Array (concatenate)(w347, w346) -> (w345:T16[])
        n229 = Bundle By Name(cluster=w341, "Script"=w345) -> (w342:T22)
      }
      event "Telescope Focus.Move Focus": Value Change {
        # "Telescope Focus"
        n230 = event-data() -> ()  [unwired: 1 in, 6 out]
        n231 = Unbundle By Name(w352) -> ("Script"=w358:T16[], "state"=w355:refnum<user-event>)
        n232 = Unbundle By Name("Telescope Focus") -> ("Position"=w350:dbl)
        n233 = Generate User Event(user event=w355, event data cluster="update script" ("event data")) -> ()  [unwired: 2 in, 2 out]
        n234 = Bundle By Name(cluster=T16 {"Action"=enum."Acquire Images", "Data"=variant}, "Action"=CC_enum_Script_Action."Telescope Move", "Data"=w350) -> (w357:T16)
        n235 = Build Array (concatenate)(w358, w357) -> (w356:T16[])
        n236 = Bundle By Name(cluster=w352, "Script"=w356) -> (w353:T22)
      }
      event "Move Telescope": Value Change {
        n237 = event-data() -> ()  [unwired: 1 in, 6 out]
        n238 = Unbundle By Name(w365) -> ("Script"=w371:T16[], "state"=w368:refnum<user-event>)
        n239 = Unbundle By Name("RA and DEC String 2") -> ("RA"=w363:string, "DEC"=w362:string)
        n240 = call "PRIME Telescope Convert HHMMSS to RA and DEC Angle.vi"("Dec String"=w362, "RA String"=w363) -> ("RA and DEC"=w361:T15)  [unwired: 7 in, 2 out]
        n241 = Generate User Event(user event=w368, event data cluster="update script" ("event data")) -> ()  [unwired: 2 in, 2 out]
        n242 = Bundle By Name(cluster=T16 {"Action"=enum."Acquire Images", "Data"=variant}, "Action"=CC_enum_Script_Action."Telescope RA DEC", "Data"=w361) -> (w370:T16)
        n243 = Build Array (concatenate)(w371, w370) -> (w369:T16[])
        n244 = Bundle By Name(cluster=w365, "Script"=w369) -> (w366:T22)
      }
      event "Relative", "Absolute": Value Change {
        n245 = event-data() -> ()  [unwired: 1 in, 6 out]
        n246 = Unbundle By Name(w386) -> ("state"=w388:refnum<user-event>, "Script"=w389:T16[])
        n247 = Bundle By Name(cluster=T26 {"Motor"=0, "Position"=0} ("Cluster"), "Motor"="Select Motor (0:n-1)", "Position"="Steps") -> (w378:T26)
        n248 = Select(t=CC_enum_Script_Action."Focus Move Absolute" ("Action"), s="Absolute", f=CC_enum_Script_Action."Telescope Home" ("Action")) -> (s? t:f=w376:T17)
        n249 = Bundle By Name(cluster=T16 {"Action"=enum."Acquire Images", "Data"=variant}, "Action"=w376, "Data"=w378) -> (w384:T16)
        n250 = Generate User Event(user event=w388, event data cluster="update script" ("event data")) -> ()  [unwired: 2 in, 2 out]
        n251 = Build Array (concatenate)(w389, w384) -> (w383:T16[])
        n252 = Bundle By Name(cluster=w386, "Script"=w383) -> (w387:T22)
      }
      event "Home": Value Change {
        n253 = event-data() -> ()  [unwired: 1 in, 6 out]
        n254 = local read "Select Motor (0:n-1)"() -> (w392:i32)
        n255 = Unbundle By Name(w390) -> ("state"=w398:refnum<user-event>, "Script"=w399:T16[])
        n256 = Bundle By Name(cluster=T16 {"Action"=enum."Acquire Images", "Data"=variant}, "Action"=CC_enum_Script_Action."Focus Set Home", "Data"=w392) -> (w396:T16)
        n257 = Generate User Event(user event=w398, event data cluster="update script" ("event data")) -> ()  [unwired: 2 in, 2 out]
        n258 = Build Array (concatenate)(w399, w396) -> (w395:T16[])
        n259 = Bundle By Name(cluster=w390, "Script"=w395) -> (w391:T22)
      }
      event "Objects": Value Change {
        n260 = event-data() -> ("CtlRef"=w408:refnum<vi>, "NewVal"=w406:i32)  [unwired: 1 in]
        n261 = property class="MCListbox (strict)"(reference=w408) -> ("ItemNames"=w407:string[][])  [unwired: 1 in, 2 out]
        n262 = Unbundle By Name(w402) -> ("state"=w401:refnum<user-event>)
        n263 = Generate User Event(user event=w401, event data cluster="show object" ("event data")) -> ()  [unwired: 2 in, 2 out]
        n264 = Index Array(array=w407, index (row)=w406, index (col)=0 ("disabled index (col)")) -> (element=w404:string)
        n265 = Bundle By Name(cluster=w402, "curr object"=w404) -> (w403:T22)
      }
      event "Obj Add/Replace": Value Change {
        n266 = event-data() -> ()  [unwired: 1 in, 1 out]
        n267 = call "CC RA and DEC to decimal.vi"("RA and DEC String"="RA and DEC String") -> ("error out"=w409:errorcluster, "RA and DEC"=w411:T15)  [unwired: 9 in]
        n268 = case shown="No Error" w409 {
          tunnel: [w417 w429] -> w413
          tunnel: w412 -> [w416 w429]
          tunnel: w411 -> [w415 _]
          frame No Error {
            n269 = Unbundle By Name(w416) -> ("state"=w420:refnum<user-event>, "Object Map"=w427:map{string, T14})
            n270 = Unbundle By Name("Object Name") -> ("Name"=w426:string)
            n271 = Bundle By Name(cluster=T14 {"Object"={"Name"=""}, "Sidereal Rate"={"dRA"=0.0, "dDEC"=0.0}, "RA and DEC"={"RA"=0.0, "DEC"=0.0}, "muRA muDEC Epoch"={"muRA"=0.0, "muDEC"=0.0, "Epoch"=0.0}, "Offsets"={"RA"=0.0, "DEC"=0.0, "ROT"=0.0}} ("value"), "Object"="Object Name", "Sidereal Rate"="Sidereal Rate", "RA and DEC"=w415, "muRA muDEC Epoch"="Proper Motion", "Offsets"="Offsets") -> (w421:T14)
            n272 = Generate User Event(user event=w420, event data cluster="show object list" ("event data")) -> ()  [unwired: 2 in, 2 out]
            n273 = Insert Into Map(map in=w427, key=w426, value=w421) -> (map out=w418:map{string, T14})  [unwired: 2 out]
            n274 = Bundle By Name(cluster=w416, "Object Map"=w418) -> (w417:T22)
          }
          frame Error {
            n275 = One Button Dialog(message="RA and/or DEC invalid format. \nRA format: HH:MM:SS.nnn\nDEC format: DEG:arcmin:arcsec.nn") -> ()  [unwired: 1 in, 1 out]
          }
        }
      }
      event "Obj Remove": Value Change {
        n276 = event-data() -> ()  [unwired: 1 in, 1 out]
        n277 = Unbundle By Name(w432) -> ("Object Map"=w442:map{string, T14}, "state"=w430:refnum<user-event>)
        n278 = property on="Objects" class="MCListbox (strict)"() -> ("ItemNames"=w444:string[][], "Value"=w437:i32)  [unwired: 2 in, 2 out]
        n279 = Generate User Event(user event=w430, event data cluster="show object list" ("event data")) -> (error out=w431:errorcluster)  [unwired: 2 in, 1 out]
        n280 = Index Array(array=w444, index (row)=w437, index (col)=0 ("disabled index (col)")) -> (element=w441:string)
        n281 = Remove From Map(10:w441, 11:w442) -> (3:w439:map{string, T14})  [unwired: 2 out]
        n282 = Collection Size(1:w439) -> (0:w436:i32)
        n283 = Bundle By Name(cluster=w432, "Object Map"=w439) -> (w433:T22)
        n284 = Greater Or Equal?(x=w436, y=w437) -> (x >= y?=w438:bool)
        n285 = Decrement(x=w436) -> (x-1=w435:i32)
        n286 = Select(t=w435, s=w438, f=w437) -> (s? t:f=w434:i32)
        n287 = property on="Objects" class="MCListbox (strict)"(error in=w431, "Val(Sgnl)"=w434) -> ()  [unwired: 1 in, 2 out]
      }
      event "Obj Add to Script": Value Change {
        n288 = event-data() -> ()  [unwired: 1 in, 6 out]
        n289 = Unbundle By Name(w447) -> ("state"=w445:refnum<user-event>, "Script"=w448:T16[], "Object Map"=w452:map{string, T14})
        n290 = property on="Objects" class="MCListbox (strict)"() -> ("ItemNames"=w455:string[][], "Value"=w454:i32)  [unwired: 2 in, 2 out]
        n291 = Index Array(array=w455, index (row)=w454, index (col)=0 ("disabled index (col)")) -> (element=w451:string)
        n292 = Look In Map(map=w452, key=w451) -> (key not found?=w450:bool, value=w449:T14)  [unwired: 1 in]
        n293 = case shown="False" w450 {
          tunnel: w449 -> [w463 _]
          tunnel: w448 -> [w461 _]
          tunnel: w447 -> [w460 w466]
          tunnel: [w458 w466] -> w446
          tunnel: w445 -> [w457 _]
          frame False {
            (unwired) T14 {"Object"={"Name"=""}, "Sidereal Rate"={"dRA"=0.0, "dDEC"=0.0}, "RA and DEC"={"RA"=0.0, "DEC"=0.0}, "muRA muDEC Epoch"={"muRA"=0.0, "muDEC"=0.0, "Epoch"=0.0}, "Offsets"={"RA"=0.0, "DEC"=0.0, "ROT"=0.0}} ("Object")
            n294 = Generate User Event(user event=w457, event data cluster="update script" ("event data")) -> ()  [unwired: 2 in, 2 out]
            n295 = Bundle By Name(cluster=T16 {"Action"=enum."Acquire Images", "Data"=variant}, "Action"=CC_enum_Script_Action."Define Object", "Data"=w463) -> (w462:T16)
            n296 = Build Array (concatenate)(w461, w462) -> (w459:T16[])
            n297 = Bundle By Name(cluster=w460, "Script"=w459) -> (w458:T22)
          }
          frame True {
            n298 = One Button Dialog(message="Add Object to List before adding to script.") -> ()  [unwired: 1 in, 1 out]
          }
        }
      }
      event "Exp Add to Script": Value Change {
        n299 = event-data() -> ()  [unwired: 1 in, 6 out]
        n300 = Unbundle By Name(w470) -> ("state"=w468:refnum<user-event>, "Script"=w471:T16[], "Exp Map"=w475:map{string, T6})
        n301 = property on="Exposures" class="MCListbox (strict)"() -> ("ItemNames"=w478:string[][], "Value"=w477:i32)  [unwired: 2 in, 2 out]
        n302 = Index Array(array=w478, index (row)=w477, index (col)=0 ("disabled index (col)")) -> (element=w474:string)
        n303 = Look In Map(map=w475, key=w474) -> (key not found?=w473:bool, value=w472:T6)  [unwired: 1 in]
        n304 = case shown="False" w473 {
          tunnel: w472 -> [w486 _]
          tunnel: w471 -> [w484 _]
          tunnel: w470 -> [w483 w489]
          tunnel: [w481 w489] -> w469
          tunnel: w468 -> [w480 _]
          frame False {
            n305 = Generate User Event(user event=w480, event data cluster="update script" ("event data")) -> ()  [unwired: 2 in, 2 out]
            n306 = Bundle By Name(cluster=T16 {"Action"=enum."Acquire Images", "Data"=variant}, "Action"=CC_enum_Script_Action."Define Exposure", "Data"=w486) -> (w485:T16)
            n307 = Build Array (concatenate)(w484, w485) -> (w482:T16[])
            n308 = Bundle By Name(cluster=w483, "Script"=w482) -> (w481:T22)
          }
          frame True {
            n309 = One Button Dialog(message="Add Object to List before adding to script.") -> ()  [unwired: 1 in, 1 out]
          }
        }
      }
      event "Dither Add to Script": Value Change {
        n310 = event-data() -> ()  [unwired: 1 in, 1 out]
        n311 = Unbundle By Name(w495) -> ("state"=w493:refnum<user-event>, "Script"=w496:T16[], "Dither Map"=w498:map{string, T19})
        n312 = property on="Dithering" class="MCListbox (strict)"() -> ("ItemNames"=w501:string[][], "Value"=w500:i32)  [unwired: 2 in, 2 out]
        n313 = Index Array(array=w501, index (row)=w500, index (col)=1 ("disabled index (col)")) -> (element=w491:string)
        n314 = Look In Map(map=w498, key=w491) -> (key not found?=w497:bool, value=w492:T19)  [unwired: 1 in]
        n315 = case shown="False" w497 {
          tunnel: w496 -> [w512 _]
          tunnel: w495 -> [w511 w524]
          tunnel: [w509 w524] -> w494
          tunnel: w493 -> [w508 _]
          tunnel: w492 -> [w506 _]
          tunnel: w491 -> [w502 _]
          frame False {
            n316 = Unbundle By Name(w506) -> ("Dithering Type"=w505:T20, "Random Dither"=w503:T8, "Dithering Offsets"=w504:T9)
            n317 = Generate User Event(user event=w508, event data cluster="update script" ("event data")) -> ()  [unwired: 2 in, 2 out]
            n318 = case shown="\"Random\", Default" w505 {
              tunnel: [w517 w522] -> w513
              tunnel: w504 -> [_ w521]
              tunnel: w503 -> [w515 _]
              tunnel: w502 -> [w514 w520]
              frame "Random", Default {
                n319 = Bundle By Name(cluster=w515, "Name"=w514) -> (w516:T8)
                n320 = Bundle By Name(cluster=T16 {"Action"=enum."Define Random Dither", "Data"=variant}, "Data"=w516) -> (w517:T16)
              }
              frame "Offsets" {
                n321 = Bundle By Name(cluster=w521, "Name"=w520) -> (w519:T9)
                n322 = Bundle By Name(cluster=T16 {"Action"=enum."Define Dithering", "Data"=variant}, "Data"=w519) -> (w522:T16)
              }
            }
            n323 = Build Array (concatenate)(w512, w513) -> (w510:T16[])
            n324 = Bundle By Name(cluster=w511, "Script"=w510) -> (w509:T22)
          }
          frame True {
            n325 = One Button Dialog(message="Add Object to List before adding to script.") -> ()  [unwired: 1 in, 1 out]
          }
        }
      }
      event "Exposures": Value Change {
        n326 = event-data() -> ("CtlRef"=w529:refnum<vi>, "NewVal"=w528:i32)  [unwired: 1 in]
        n327 = property class="MCListbox (strict)"(reference=w529) -> ("ItemNames"=w534:string[][])  [unwired: 1 in, 2 out]
        n328 = Unbundle By Name(w526) -> ("state"=w531:refnum<user-event>)
        n329 = Generate User Event(user event=w531, event data cluster="show exp" ("event data")) -> ()  [unwired: 2 in, 2 out]
        n330 = Index Array(array=w534, index (row)=w528, index (col)=0 ("disabled index (col)")) -> (element=w532:string)
        n331 = Bundle By Name(cluster=w526, "curr object"=w532) -> (w527:T22)
      }
      event "Exp Add/Replace": Value Change {
        n332 = event-data() -> ()  [unwired: 1 in, 6 out]
        n333 = Unbundle By Name(w537) -> ("state"=w536:refnum<user-event>, "Exp Map"=w542:map{string, T6})
        n334 = Unbundle By Name("Exposure") -> ("Name"=w541:string)
        n335 = Insert Into Map(map in=w542, key=w541, value="Exposure") -> (map out=w539:map{string, T6})  [unwired: 2 out]
        n336 = Generate User Event(user event=w536, event data cluster="show exp list" ("event data")) -> ()  [unwired: 2 in, 2 out]
        n337 = Bundle By Name(cluster=w537, "Exp Map"=w539) -> (w538:T22)
      }
      event "Exp Remove": Value Change {
        n338 = event-data() -> ()  [unwired: 1 in, 6 out]
        n339 = Unbundle By Name(w543) -> ("Exp Map"=w555:map{string, T6}, "state"=w545:refnum<user-event>)
        n340 = property on="Exposures" class="MCListbox (strict)"() -> ("ItemNames"=w557:string[][], "Value"=w550:i32)  [unwired: 2 in, 2 out]
        n341 = Generate User Event(user event=w545, event data cluster="show exp list" ("event data")) -> (error out=w546:errorcluster)  [unwired: 2 in, 1 out]
        n342 = Index Array(array=w557, index (row)=w550, index (col)=0 ("disabled index (col)")) -> (element=w554:string)
        n343 = Remove From Map(10:w554, 11:w555) -> (3:w552:map{string, T6})  [unwired: 2 out]
        n344 = Collection Size(1:w552) -> (0:w549:i32)
        n345 = Bundle By Name(cluster=w543, "Exp Map"=w552) -> (w544:T22)
        n346 = Greater Or Equal?(x=w549, y=w550) -> (x >= y?=w551:bool)
        n347 = Decrement(x=w549) -> (x-1=w548:i32)
        n348 = Select(t=w548, s=w551, f=w550) -> (s? t:f=w547:i32)
        n349 = property on="Exposures" class="MCListbox (strict)"(error in=w546, "Val(Sgnl)"=w547) -> ()  [unwired: 1 in, 2 out]
      }
      event "Dithering": Value Change {
        n350 = event-data() -> ("CtlRef"=w561:refnum<vi>, "NewVal"=w560:i32)  [unwired: 1 in, 4 out]
        n351 = property class="MCListbox (strict)"(reference=w561) -> ("ItemNames"=w566:string[][])  [unwired: 1 in, 2 out]
        n352 = Unbundle By Name(w558) -> ("state"=w563:refnum<user-event>)
        n353 = Generate User Event(user event=w563, event data cluster="show dither" ("event data")) -> ()  [unwired: 2 in, 2 out]
        n354 = Index Array(array=w566, index (row)=w560, index (col)=1 ("disabled index (col)")) -> (element=w564:string)
        n355 = Bundle By Name(cluster=w558, "curr object"=w564) -> (w559:T22)
      }
      event "Dithering Add/Replace": Value Change {
        n356 = event-data() -> ()  [unwired: 1 in, 6 out]
        n357 = case shown="\"Offset\"" "Dither Select" {
          tunnel: [w581 w592] -> w573
          tunnel: w572 -> [w580 w591]
          tunnel: "Name" -> [w577 w589]
          tunnel: [w576 w588] -> w568
          tunnel: T19 {"Name"="", "Dithering Offsets"={"Name"="", "Dithering Offsets"={"Offsets"=[]}}, "Dithering Type"=enum."Random", "Random Dither"={"Count"=1, "Radius"=1.0, "Name"=""}} ("value") -> [w575 w586]
          frame "Random", Default {
            n358 = Unbundle By Name(w580) -> ("state"=w583:refnum<user-event>, "Dither Map"=w584:map{string, T19})
            n359 = Bundle By Name(cluster=w575, "Name"=w577, "Dithering Type"=CC_enum_Dithering_Types."Random", "Random Dither"="Random Dither") -> (w574:T19)
            n360 = Insert Into Map(map in=w584, key=w577, value=w574) -> (map out=w576:map{string, T19})  [unwired: 2 out]
            n361 = Generate User Event(user event=w583, event data cluster="show dither list" ("event data")) -> ()  [unwired: 2 in, 2 out]
            n362 = Bundle By Name(cluster=w580, "Dither Map"=w576) -> (w581:T22)
          }
          frame "Offset" {
            n363 = Unbundle By Name(w591) -> ("state"=w594:refnum<user-event>, "Dither Map"=w595:map{string, T19})
            n364 = Bundle By Name(cluster=w586, "Name"=w589, "Dithering Type"=CC_enum_Dithering_Types."Offsets", "Dithering Offsets"="Dithering Offset") -> (w585:T19)
            n365 = Generate User Event(user event=w594, event data cluster="show dither list" ("event data")) -> ()  [unwired: 2 in, 2 out]
            n366 = Insert Into Map(map in=w595, key=w589, value=w585) -> (map out=w588:map{string, T19})  [unwired: 2 out]
            n367 = Bundle By Name(cluster=w591, "Dither Map"=w588) -> (w592:T22)
          }
        }
        n368 = call "CC Rd Wr Dither Map.vi"("Write? (F:Read)"=TRUE, "Dither Map"=w568) -> ()  [unwired: 8 in, 2 out]
      }
      event "Dithering Remove": Value Change {
        n369 = event-data() -> ()  [unwired: 1 in, 6 out]
        n370 = Unbundle By Name(w609) -> ("Dither Map"=w608:map{string, T19}, "state"=w611:refnum<user-event>)
        n371 = property on="Dither Select" class="TabCtl (strict)" props=["Value"]() -> ()  [unwired: 2 in, 3 out]
        n372 = property on="Dithering" class="MCListbox (strict)"() -> ("ItemNames"=w607:string[][], "Value"=w602:i32)  [unwired: 2 in, 2 out]
        n373 = Index Array(array=w607, index (row)=w602, index (col)=1 ("disabled index (col)")) -> (element=w605:string)
        n374 = Generate User Event(user event=w611, event data cluster="show dither list" ("event data")) -> (error out=w598:errorcluster)  [unwired: 2 in, 1 out]
        n375 = Remove From Map(10:w605, 11:w608) -> (3:w596:map{string, T19})  [unwired: 2 out]
        n376 = Collection Size(1:w596) -> (0:w601:i32)
        n377 = Greater Or Equal?(x=w601, y=w602) -> (x >= y?=w603:bool)
        n378 = Bundle By Name(cluster=w609, "Dither Map"=w596) -> (w610:T22)
        n379 = Decrement(x=w601) -> (x-1=w600:i32)
        n380 = Select(t=w600, s=w603, f=w602) -> (s? t:f=w599:i32)
        n381 = call "CC Rd Wr Dither Map.vi"("Write? (F:Read)"=TRUE, "Dither Map"=w596) -> ()  [unwired: 8 in, 2 out]
        n382 = property on="Dithering" class="MCListbox (strict)"(error in=w598, "Val(Sgnl)"=w599) -> ()  [unwired: 1 in, 2 out]
      }
      event "Add FW 1", "Add FW 2", "Add FW 3", "Add FW 4": Value Change {
        # "MoveFilterWheel\nSyntax:\nMoveFilterWheel Wheel1:n,Wheel2:n\nParameter\tUnits\tPurpose\nWheel1\t\tPosition of Wheel one (integer)\nWheel2\t\tPosition of Wheel two (integer)"
        n383 = event-data() -> ("CtlRef"=w629:refnum<vi>)  [unwired: 1 in, 2 out]
        n384 = property class="Bool"(reference=w629) -> ("Label.Text"=w628:string)  [unwired: 1 in, 2 out]
        n385 = Unbundle By Name(w615) -> ("state"=w617:refnum<user-event>, "Script"=w616:T16[])
        n386 = Build Array("Filter Wheel 1", "Filter Wheel 2", "Filter Wheel 3", "Filter Wheel 4") -> (w621:i32[])
        n387 = Match Pattern(string=w628, regular expression="Add FW ") -> (after substring=w626:string)  [unwired: 1 in, 3 out]
        n388 = Decimal String To Number(string=w626) -> (number=w620:i32)  [unwired: 2 in, 1 out]
        n389 = Decrement(x=w620) -> (x-1=w612:i32)
        n390 = Index Array(array=w621, index=w612) -> (element=w619:i32)
        n391 = Bundle By Name(cluster=T27 {"Wheel"=0, "Filter"=0} ("Acquire Parameters in"), "Wheel"=w612, "Filter"=w619) -> (w618:T27)
        n392 = Generate User Event(user event=w617, event data cluster="update script" ("event data")) -> ()  [unwired: 2 in, 2 out]
        n393 = Bundle By Name(cluster=T16 {"Action"=enum."Acquire Images", "Data"=variant}, "Action"=CC_enum_Script_Action."Set Filter Wheel", "Data"=w618) -> (w632:T16)
        n394 = Build Array (concatenate)(w616, w632) -> (w631:T16[])
        n395 = Bundle By Name(cluster=w615, "Script"=w631) -> (w614:T22)
      }
      event "Tab Control": Value Change {
        n396 = event-data() -> ("NewVal"=w637:T1)  [unwired: 1 in]
        n397 = case shown="\"Setup\", Default" w637 {
          tunnel: w636 -> [_ _ w666 w672]
          tunnel: "Script" -> [_ _ _ w670]
          frame "Setup", Default {
          }
          frame "Acquire" {
            w638 = refnum<vi> refnum  # ComboBox
            n398 = property on="Objects" class="MCListbox (strict)"() -> ("ItemNames"=w663:string[][], "Value"=w657:i32)  [unwired: 2 in, 2 out]
            n399 = property on="Exposures" class="MCListbox (strict)"() -> ("ItemNames"=w648:string[][], "Value"=w647:i32)  [unwired: 2 in, 2 out]
            n400 = property on="Dithering" class="MCListbox (strict)"() -> ("ItemNames"=w649:string[][], "Value"=w646:i32)  [unwired: 2 in, 2 out]
            n401 = property on="Acquire Parameters" class="Clust (strict)"() -> ("Controls[]"=w662:refnum<vi>[])  [unwired: 2 in, 2 out]
            n402 = Index Array(array=w663, index (col)=0 ("disabled index (col)")) -> (element=w658:string[])  [unwired: 1 in]
            n403 = Index Array(array=w648, index (col)=0 ("disabled index (col)")) -> (element=w654:string[])  [unwired: 1 in]
            n404 = Index Array(array=w649, index (col)=1 ("disabled index (col)")) -> (element=w651:string[])  [unwired: 1 in]
            n405 = Index Array(array=w658, index=w657) -> (element=w656:string)
            n406 = Index Array(array=w654, index=w647) -> (element=w655:string)
            n407 = Index Array(array=w662) -> (element #1=w661:refnum<vi>, element #2=w643:refnum<vi>, element #3=w640:refnum<vi>)  [unwired: 3 in]
            n408 = Index Array(array=w651, index=w646) -> (element=w650:string)
            n409 = To More Specific Class(target class=w638, reference=w661) -> (specific class reference=w660:refnum<vi>, error out=w639:errorcluster)  [unwired: 1 in]
            n410 = To More Specific Class(target class=w638, reference=w643) -> (specific class reference=w645:refnum<vi>, error out=w644:errorcluster)  [unwired: 1 in]
            n411 = To More Specific Class(target class=w638, reference=w640) -> (specific class reference=w642:refnum<vi>, error out=w641:errorcluster)  [unwired: 1 in]
            n412 = property class="CmbBox"(reference=w660, error in=w639, "Strings[]"=w658, "Value"=w656) -> ()  [unwired: 2 out]
            n413 = property class="CmbBox"(reference=w645, error in=w644, "Strings[]"=w654, "Value"=w655) -> ()  [unwired: 2 out]
            n414 = property class="CmbBox"(reference=w642, error in=w641, "Strings[]"=w651, "Value"=w650) -> ()  [unwired: 2 out]
          }
          frame "Text" {
            n415 = Unbundle By Name(w666) -> ("Script"=w665:T16[])
            n416 = call "CC Generate Script Text.vi"("Script"=w665) -> ("Script String"=→"Script As Text":string)  [unwired: 9 in, 1 out]
          }
          frame "Test" {
            n417 = Unbundle By Name(w672) -> ("Script"=w671:T16[])
            n418 = Index Array(array=w671, index=w670) -> (element=w669:T16)
            n419 = Build Array(w669) -> (w668:T16[])
            n420 = call "CC Generate Script Text.vi"("Script"=w668) -> ("Script String"=w667:string)  [unwired: 9 in, 1 out]
            n421 = property on="Script Line" class="Str"("Value"=w667) -> ()  [unwired: 2 in, 2 out]
          }
        }
      }
      event "Add Image Acq": Value Change {
        n422 = event-data() -> ()  [unwired: 1 in, 6 out]
        n423 = Unbundle By Name(w675) -> ("Script"=w679:T16[], "state"=w674:refnum<user-event>)
        n424 = Generate User Event(user event=w674, event data cluster="update script" ("event data")) -> ()  [unwired: 2 in, 2 out]
        n425 = Bundle By Name(cluster=T16 {"Action"=enum."Acquire Images", "Data"=variant}, "Action"=CC_enum_Script_Action."Acquire Images", "Data"="Acquire Parameters") -> (w678:T16)
        n426 = Build Array (concatenate)(w679, w678) -> (w677:T16[])
        n427 = Bundle By Name(cluster=w675, "Script"=w677) -> (w676:T22)
      }
      event "New Button": Value Change {
        n428 = event-data() -> ()  [unwired: 1 in, 6 out]
        n429 = Unbundle By Name(w686) -> ("state"=w685:refnum<user-event>)
        n430 = call "Script Name2"() -> ("Script Name"=w684:string, "OK"=w683:bool)  [unwired: 17 in, 1 out]
        n431 = case shown="True" w683 {
          tunnel: [w688 w696] -> w687
          tunnel: w686 -> [w688 w695]
          tunnel: w685 -> [_ w694]
          tunnel: w684 -> [_ w692]
          frame False {
          }
          frame True {
            n432 = property on="Script Name" class="Ring (strict)"() -> ("Strings []"=w690:string[])  [unwired: 2 in, 2 out]
            n433 = Generate User Event(user event=w694, event data cluster="update script" ("event data")) -> ()  [unwired: 2 in, 2 out]
            n434 = Build Array (concatenate)(w690, w692) -> (w691:string[])
            n435 = Array Size(array=w690) -> (size(s)=w689:i32)
            n436 = Bundle By Name(cluster=w695, "Settings.Script"=w692, "Script"=T16[] []) -> (w696:T22)
            n437 = property on="Script Name" class="Ring (strict)"("Strings []"=w691, "Value"=w689) -> ()  [unwired: 2 in, 2 out]
          }
        }
      }
      event "Save Script": Value Change {
        n438 = event-data() -> ()  [unwired: 1 in, 6 out]
        n439 = Unbundle By Name(w698) -> ("state"=w700:refnum<user-event>)
        n440 = Generate User Event(user event=w700, event data cluster="save script" ("event data")) -> ()  [unwired: 2 in, 2 out]
      }
      event "Save As Button": Value Change {
        n441 = event-data() -> ()  [unwired: 1 in, 6 out]
        n442 = call "Script Name"() -> ("Script Name"=w701:string, "OK"=w705:bool)  [unwired: 17 in, 1 out]
        n443 = Unbundle By Name(w703) -> ("state"=w704:refnum<user-event>)
        n444 = case shown="True" w705 {
          tunnel: w704 -> [_ w711]
          tunnel: w703 -> [w706 w707]
          tunnel: [w706 w708] -> w702
          tunnel: w701 -> [_ w709]
          frame False {
          }
          frame True {
            n445 = Bundle By Name(cluster=w707, "Settings.Script"=w709) -> (w708:T22)
            n446 = Generate User Event(user event=w711, event data cluster="save script" ("event data")) -> ()  [unwired: 2 in, 2 out]
          }
        }
      }
      event "Delete": Value Change {
        n447 = event-data() -> ()  [unwired: 1 in, 6 out]
        n448 = Unbundle By Name(w714) -> ("state"=w713:refnum<user-event>)
        n449 = Generate User Event(user event=w713, event data cluster="delete script" ("event data")) -> ()  [unwired: 2 in, 2 out]
      }
      event "Script Name": Value Change {
        n450 = event-data() -> ("NewVal"=w716:u16)  [unwired: 1 in]
        n451 = Unbundle By Name(w720) -> ("state"=w719:refnum<user-event>)
        n452 = property on="Script Name" class="Ring (strict)"() -> ("Strings []"=w717:string[])  [unwired: 2 in, 2 out]
        n453 = Generate User Event(user event=w719, event data cluster="load script" ("event data")) -> ()  [unwired: 2 in, 2 out]
        n454 = Index Array(array=w717, index=w716) -> (element=w715:string)
        n455 = Bundle By Name(cluster=w720, "Settings.Script"=w715) -> (w721:T22)
      }
      event "Script": Double Click {
        n456 = event-data() -> ("Row"=w726:i32)  [unwired: 1 in]
        n457 = Unbundle By Name(w728) -> ("Script"=w727:T16[])
        n458 = Index Array(array=w727, index=w726) -> (element=w725:T16)
        n459 = Unbundle By Name(w725) -> ("Action"=w724:T17, "Data"=w723:variant)
        n460 = case shown="\"Define Object\"" w724 {
          tunnel: [T28."Noop" ("Value (Signaling)") T28."Object" ("Value (Signaling)") T29."Exposure" ("Value (Signaling)") T28."Dithering" ("Value (Signaling)") u32 0 ("Value (Signaling)") T28."Acquire" ("Value (Signaling)") T28."Filter Wheel" ("Value (Signaling)") T31."Telescope" ("Value (Signaling)") T28."Focus" ("Value (Signaling)") T28."Focus" ("Value (Signaling)") T28."Macro" ("Value (Signaling)") T28."Pause" ("Value (Signaling)") T28."Ask" ("Value (Signaling)") T28."Dithering" ("Value (Signaling)") u32 0 ("Value (Signaling)")] -> w722
          tunnel: w723 -> [_ w741 w745 w750 _ w755 _ _ _ _ _ w765 w769 w772 _]
          frame "Noop", Default {
          }
          frame "Define Object" {
            (unwired) T44."Object" ("Value (Signaling)")
            n461 = Variant To Data(type=T14 {"Object"={"Name"=""}, "Sidereal Rate"={"dRA"=0.0, "dDEC"=0.0}, "RA and DEC"={"RA"=0.0, "DEC"=0.0}, "muRA muDEC Epoch"={"muRA"=0.0, "muDEC"=0.0, "Epoch"=0.0}, "Offsets"={"RA"=0.0, "DEC"=0.0, "ROT"=0.0}} ("Object"), Variant=w741) -> (data=w739:T14)  [unwired: 1 in, 1 out]
            n462 = Unbundle By Name(w739) -> ("Object"=w730:cluster{"Name":string}, "Sidereal Rate"=w738:T3, "RA and DEC"=w733:T15, "muRA muDEC Epoch"=w737:T4, "Offsets"=w736:T5)
            n463 = call "CC Convert RA and DEC to HHMMSS.vi"("RA and DEC"=w733) -> ("DEC String"=w732:string, "RA String"=w735:string)  [unwired: 9 in]
            n464 = property on="Offsets" class="Clust (strict)"("Val(Sgnl)"=w736) -> ()  [unwired: 2 in, 2 out]
            n465 = property on="muRA muDEC" class="Clust (strict)"("Val(Sgnl)"=w737) -> ()  [unwired: 2 in, 2 out]
            n466 = property on="Object Name" class="Clust (strict)"("Val(Sgnl)"=w730) -> ()  [unwired: 2 in, 2 out]
            n467 = property on="Sidereal Rate" class="Clust (strict)"("Val(Sgnl)"=w738) -> ()  [unwired: 2 in, 2 out]
            n468 = Bundle("RA String"=w735, "DEC String"=w732) -> (w734:cluster{"RA String":string, "DEC String":string})  [unwired: 1 in]
            n469 = local write "RA and DEC String"(w734) -> ()
          }
          frame "Define Exposure" {
            n470 = Variant To Data(type=T6 {"Mode"=enum."CDS", "Integration Time"=1.0, "Name"="", "Images"=1} ("Exposure"), Variant=w745) -> (data=w743:T6)  [unwired: 1 in, 1 out]
            n471 = property on="Exposure" class="Clust (strict)"("Val(Sgnl)"=w743) -> ()  [unwired: 2 in, 2 out]
          }
          frame "Define Dithering" {
            n472 = Variant To Data(type=T9 {"Name"="", "Dithering Offsets"={"Offsets"=[]}} ("Dithering Offsets"), Variant=w750) -> (data=w746:T9)  [unwired: 1 in, 1 out]
            n473 = Unbundle By Name(w746) -> ("Name"=w748:string)
            n474 = property on="Dithering Offset" class="Clust (strict)"("Val(Sgnl)"=w746) -> ()  [unwired: 2 in, 2 out]
            n475 = property on="Name" class="Str"("Value"=w748) -> ()  [unwired: 2 in, 2 out]
          }
          frame "Telescope Move" {
          }
          frame "Acquire Images" {
            n476 = Variant To Data(type=T30 {"Object"="", "Exposure"="", "Dithering"=""} ("Acquire Parameters"), Variant=w755) -> (data=w753:T30)  [unwired: 1 in, 1 out]
            n477 = property on="Acquire Parameters" class="Clust (strict)"("Val(Sgnl)"=w753) -> ()  [unwired: 2 in, 2 out]
          }
          frame "Set Filter Wheel" {
          }
          frame "Telescope Home" {
          }
          frame "Focus Move Absolute" {
          }
          frame "Focus Set Home" {
          }
          frame "Macro" {
          }
          frame "Pause" {
            n478 = Variant To Data(type=T32 {"Time (s)"=0.0} ("Pause Parameters"), Variant=w765) -> (data=w763:T32)  [unwired: 1 in, 1 out]
            n479 = Unbundle By Name(w763) -> ("Time (s)"=w762:dbl)
            n480 = property on="Seconds to Pause" class="DigNum (strict)"("Val(Sgnl)"=w762) -> ()  [unwired: 2 in, 2 out]
          }
          frame "Ask User" {
            n481 = Variant To Data(type="", Variant=w769) -> (data=w767:string)  [unwired: 1 in, 1 out]
            n482 = property on="Message for User" class="Str"("Val(Sgnl)"=w767) -> ()  [unwired: 2 in, 2 out]
          }
          frame "Define Random Dither" {
            n483 = Variant To Data(type=T8 {"Count"=1, "Radius"=1.0, "Name"=""} ("Dithering Offsets"), Variant=w772) -> (data=w771:T8)  [unwired: 1 in, 1 out]
            n484 = Unbundle By Name(w771) -> ("Name"=w770:string)
            n485 = property on="Random Dither" class="Clust (strict)"("Value"=w771) -> ()  [unwired: 2 in, 2 out]
            n486 = property on="Name" class="Str"("Value"=w770) -> ()  [unwired: 2 in, 2 out]
          }
          frame "Focus Move Relative" {
          }
        }
        n487 = property on="Tab Control" class="TabCtl (strict)"("Val(Sgnl)"=w722) -> ()  [unwired: 2 in, 2 out]
      }
      event "Script": Value Change {
        (unwired) T1."Telescope" ("Tab Control")
        n488 = event-data() -> ("NewVal"=w783:i32)  [unwired: 1 in]
        n489 = Unbundle By Name(w779) -> ("state"=w777:refnum<user-event>, "Script"=w786:T16[])
        n490 = Index Array(array=w786, index=w783) -> (element=w782:T16)
        n491 = Unbundle By Name(w782) -> ("Action"=w781:T17, "Data"=w780:variant)
        n492 = Build Array(w782) -> (w785:T16[])
        n493 = call "CC Generate Script Text.vi"("Script"=w785) -> ("Script String"=w784:string)  [unwired: 9 in, 1 out]
        n494 = case shown="\"Telescope RA DEC\"" w781 {
          tunnel: w780 -> [_ w797 w806 w815 w820 w825 w831 w838 w845 w849 w856 w862 w867 _ w875 w884]
          tunnel: w779 -> [w788 w793 w803 w812 w817 w822 w832 w839 w846 w850 w857 w863 w868 w870 w872 w882]
          tunnel: [w788 w792 w802 w811 w817 w822 w832 w839 w846 w850 w857 w863 w868 w870 w872 w882] -> w778
          tunnel: w777 -> [_ w791 w801 w810 _ _ _ _ _ _ _ _ _ _ _ _]
          tunnel: [w787 T1."Object" ("Tab Control") T1."Dithering" ("Tab Control") T1."Dithering" ("Tab Control") T1."Exposure" ("Tab Control") T1."Acquire" ("Tab Control") T1."Filter Wheel" ("Tab Control") T1."Telescope" ("Tab Control") T1."Telescope" ("Tab Control") T1."Telescope" ("Tab Control") T1."Macro" ("Tab Control") T1."Pause" ("Tab Control") T1."Ask" ("Tab Control") T1."Telescope" ("Tab Control") T1."Telescope" ("Tab Control") T1."Telescope" ("Tab Control")] -> w776
          frame "Noop", Default {
            n495 = property on="Tab Control" class="TabCtl (strict)"() -> ("Value"=w787:T1)  [unwired: 2 in, 2 out]
          }
          frame "Define Object" {
            n496 = Variant To Data(type=T14 {"Object"={"Name"=""}, "Sidereal Rate"={"dRA"=0.0, "dDEC"=0.0}, "RA and DEC"={"RA"=0.0, "DEC"=0.0}, "muRA muDEC Epoch"={"muRA"=0.0, "muDEC"=0.0, "Epoch"=0.0}, "Offsets"={"RA"=0.0, "DEC"=0.0, "ROT"=0.0}} ("Object"), Variant=w797) -> (data=w795:T14)  [unwired: 1 in, 1 out]
            n497 = Unbundle By Name(w795) -> ("Object.Name"=w794:string)
            n498 = Generate User Event(user event=w791, event data cluster="show object" ("event data")) -> ()  [unwired: 2 in, 2 out]
            n499 = Bundle By Name(cluster=w793, "curr object"=w794) -> (w792:T22)
          }
          frame "Define Dithering" {
            n500 = Variant To Data(type=T9 {"Name"="", "Dithering Offsets"={"Offsets"=[]}} ("Dithering Offsets"), Variant=w806) -> (data=w805:T9)  [unwired: 1 in, 1 out]
            n501 = Unbundle By Name(w805) -> ("Name"=w804:string)
            n502 = Generate User Event(user event=w801, event data cluster="show dither" ("event data")) -> ()  [unwired: 2 in, 2 out]
            n503 = Bundle By Name(cluster=w803, "curr object"=w804) -> (w802:T22)
          }
          frame "Define Random Dither" {
            n504 = Variant To Data(type=T8 {"Count"=1, "Radius"=1.0, "Name"=""} ("Dithering Offsets"), Variant=w815) -> (data=w814:T8)  [unwired: 1 in, 1 out]
            n505 = Unbundle By Name(w814) -> ("Name"=w813:string)
            n506 = Generate User Event(user event=w810, event data cluster="show dither" ("event data")) -> ()  [unwired: 2 in, 2 out]
            n507 = Bundle By Name(cluster=w812, "curr object"=w813) -> (w811:T22)
          }
          frame "Define Exposure" {
            n508 = Variant To Data(type=T6 {"Mode"=enum."CDS", "Integration Time"=1.0, "Name"="", "Images"=1} ("Exposure"), Variant=w820) -> (data=w818:T6)  [unwired: 1 in, 1 out]
            n509 = property on="Exposure" class="Clust (strict)"("Value"=w818) -> ()  [unwired: 2 in, 2 out]
          }
          frame "Acquire Images" {
            n510 = Variant To Data(type=T30 {"Object"="", "Exposure"="", "Dithering"=""} ("Acquire Parameters"), Variant=w825) -> (data=w823:T30)  [unwired: 1 in, 1 out]
            n511 = property on="Acquire Parameters" class="Clust (strict)"("Value"=w823) -> ()  [unwired: 2 in, 2 out]
          }
          frame "Set Filter Wheel" {
            n512 = Variant To Data(type=T27 {"Wheel"=0, "Filter"=0} ("Acquire Parameters"), Variant=w831) -> (data=w829:T27)  [unwired: 1 in, 1 out]
            n513 = Unbundle By Name(w829) -> ("Wheel"=w828:i32, "Filter"=w827:i32)
            n514 = case shown="0, Default" w828 {
              tunnel: w827 -> [w833 w834]
              frame 0, Default {
                n515 = property on="Filter Wheel 1" class="LstBox (strict)"("Value"=w833) -> ()  [unwired: 2 in, 2 out]
              }
              frame 1 {
                n516 = property on="Filter Wheel 2" class="LstBox (strict)"("Value"=w834) -> ()  [unwired: 2 in, 2 out]
              }
            }
          }
          frame "Focus Move Relative" {
            n517 = Variant To Data(type=0, Variant=w838) -> (data=w836:i32)  [unwired: 1 in, 1 out]
            n518 = local write "Select Motor (0:n-1)"(w836) -> ()
          }
          frame "Focus Move Absolute" {
            n519 = Variant To Data(type=T26 {"Motor"=0, "Position"=0} ("Cluster"), Variant=w845) -> (data=w843:T26)  [unwired: 1 in, 1 out]
            n520 = Unbundle By Name(w843) -> ("Motor"=w842:i32, "Position"=w841:i32)
            n521 = local write "Select Motor (0:n-1)"(w842) -> ()
            n522 = local write "Steps"(w841) -> ()
          }
          frame "Focus Set Home" {
            n523 = Variant To Data(type=0, Variant=w849) -> ()  [unwired: 1 in, 2 out]
          }
          frame "Macro" {
            n524 = Variant To Data(type="", Variant=w856) -> (data=w853:string)  [unwired: 1 in, 1 out]
            n525 = property on="Script to Call" class="Ring (strict)"() -> ("Strings []"=w854:string[])  [unwired: 2 in, 2 out]
            n526 = Search 1D Array(1D array=w854, element=w853) -> (index of element=w852:i32)  [unwired: 1 in]
            n527 = property on="Script to Call" class="Ring (strict)"("Value"=w852) -> ()  [unwired: 2 in, 2 out]
          }
          frame "Pause" {
            n528 = Variant To Data(type=T32 {"Time (s)"=0.0} ("Pause Parameters"), Variant=w862) -> (data=w861:T32)  [unwired: 1 in, 1 out]
            n529 = Unbundle By Name(w861) -> ("Time (s)"=w859:dbl)
            n530 = local write "Seconds to Pause"(w859) -> ()
          }
          frame "Ask User" {
            n531 = Variant To Data(type="", Variant=w867) -> (data=w865:string)  [unwired: 1 in, 1 out]
            n532 = local write "Message for User"(w865) -> ()
          }
          frame "Telescope Home" {
          }
          frame "Telescope Move" {
            n533 = Variant To Data(type=0.0, Variant=w875) -> (data=w873:dbl)  [unwired: 1 in, 1 out]
            n534 = property on="Position" class="DigNum (strict)"("Value"=w873) -> ()  [unwired: 2 in, 2 out]
          }
          frame "Telescope RA DEC" {
            n535 = Variant To Data(type=T15 {"RA"=0.0, "DEC"=0.0} ("Position"), Variant=w884) -> (data=w880:T15)  [unwired: 1 in, 1 out]
            n536 = call "CC Convert RA and DEC to HHMMSS.vi"("RA and DEC"=w880) -> ("DEC String"=w877:string, "RA String"=w878:string)  [unwired: 9 in]
            n537 = Bundle(cluster=cluster{"RA":string, "DEC":string} {"RA"="02:22:00.0", "DEC"="24:55:00.0"} ("RA and DEC String 2"), "RA"=w878, "DEC"=w877) -> (w876:cluster{"RA":string, "DEC":string})
            n538 = property on="RA and DEC String 2" class="Clust (strict)"("Value"=w876) -> ()  [unwired: 2 in, 2 out]
          }
        }
        n539 = property on="Script Line" class="Str"("Value"=w784) -> ()  [unwired: 2 in, 2 out]
        n540 = property on="Tab Control" class="TabCtl (strict)"("Value"=w776) -> ()  [unwired: 2 in, 2 out]
      }
      event "Send": Value Change {
        n541 = event-data() -> ()  [unwired: 1 in, 6 out]
        n542 = call "CC Script Parse.vi"("Script text"="Script Line") -> ("Syntax Errors"=w885:string, "Script Ok?"=w888:bool, "Script steps"=w889:T16[])  [unwired: 7 in, 1 out]
        n543 = case shown="True" w888 {
          tunnel: w889 -> [_ w899]
          tunnel: w886 -> [w894 w897]
          tunnel: [w894 w898] -> w887
          tunnel: w885 -> [w892 _]
          frame False {
            n544 = Format Into String(format string="Error in script line: %s", w892) -> (resulting string=w891:string)  [unwired: 2 in, 1 out]
            n545 = One Button Dialog(message=w891) -> ()  [unwired: 1 in, 1 out]
          }
          frame True {
            n546 = Bundle By Name(cluster=w897, "test"=w899) -> (w898:T22)
            n547 = Unbundle By Name(w897) -> ("state"=w896:refnum<user-event>)
            n548 = Generate User Event(user event=w896, event data cluster="run test" ("event data")) -> ()  [unwired: 2 in, 2 out]
          }
        }
      }
      event "Add Ask": Value Change {
        n549 = event-data() -> ()  [unwired: 1 in, 1 out]
        n550 = Unbundle By Name(w900) -> ("Script"=w907:T16[], "state"=w904:refnum<user-event>)
        n551 = Generate User Event(user event=w904, event data cluster="update script" ("event data")) -> ()  [unwired: 2 in, 2 out]
        n552 = Bundle By Name(cluster=T16 {"Action"=enum."Acquire Images", "Data"=variant}, "Action"=CC_enum_Script_Action."Ask User", "Data"="Message for User") -> (w906:T16)
        n553 = Build Array (concatenate)(w907, w906) -> (w905:T16[])
        n554 = Bundle By Name(cluster=w900, "Script"=w905) -> (w901:T22)
      }
      event "Add Macro": Value Change {
        n555 = event-data() -> ()  [unwired: 1 in, 1 out]
        n556 = property on="Script to Call" class="Ring (strict)"() -> ("Strings []"=w912:string[])  [unwired: 2 in, 2 out]
        n557 = Unbundle By Name(w913) -> ("Script"=w919:T16[], "state"=w916:refnum<user-event>)
        n558 = Index Array(array=w912, index="Script to Call") -> (element=w910:string)
        n559 = Generate User Event(user event=w916, event data cluster="update script" ("event data")) -> ()  [unwired: 2 in, 2 out]
        n560 = Bundle By Name(cluster=T16 {"Action"=enum."Acquire Images", "Data"=variant}, "Action"=CC_enum_Script_Action."Macro", "Data"=w910) -> (w918:T16)
        n561 = Build Array (concatenate)(w919, w918) -> (w917:T16[])
        n562 = Bundle By Name(cluster=w913, "Script"=w917) -> (w914:T22)
      }
      event "Add No-op": Value Change {
        n563 = event-data() -> ()  [unwired: 1 in, 1 out]
        n564 = Unbundle By Name(w922) -> ("Script"=w928:T16[], "state"=w925:refnum<user-event>)
        n565 = Generate User Event(user event=w925, event data cluster="update script" ("event data")) -> ()  [unwired: 2 in, 2 out]
        n566 = Bundle By Name(cluster=T16 {"Action"=enum."Acquire Images", "Data"=variant}, "Action"=CC_enum_Script_Action."Noop") -> (w927:T16)
        n567 = Build Array (concatenate)(w928, w927) -> (w926:T16[])
        n568 = Bundle By Name(cluster=w922, "Script"=w926) -> (w923:T22)
      }
      event "Add Pause": Value Change {
        n569 = event-data() -> ()  [unwired: 1 in, 1 out]
        n570 = Unbundle By Name(w934) -> ("Script"=w940:T16[], "state"=w937:refnum<user-event>)
        n571 = Bundle By Name(cluster=T32 {"Time (s)"=0.0} ("Pause Parameters"), "Time (s)"="Seconds to Pause") -> (w932:T32)
        n572 = Generate User Event(user event=w937, event data cluster="update script" ("event data")) -> ()  [unwired: 2 in, 2 out]
        n573 = Bundle By Name(cluster=T16 {"Action"=enum."Acquire Images", "Data"=variant}, "Action"=CC_enum_Script_Action."Pause", "Data"=w932) -> (w939:T16)
        n574 = Build Array (concatenate)(w940, w939) -> (w938:T16[])
        n575 = Bundle By Name(cluster=w934, "Script"=w938) -> (w935:T22)
      }
      event "Script": Shortcut Menu Activation? {
        n576 = event-data() -> ("CtlRef"=w948:refnum<vi>, "Coords"=w947:T42)  [unwired: 1 in]
        n577 = invoke class="MCListbox (strict)" method="Point To Row Column"(reference=w948, "Point"=w947) -> ("InBounds"=w945:bool, "CellPosition"=w946:T43)  [unwired: 5 in, 5 out]
        n578 = Unbundle By Name(w946) -> ("Row"=w943:i32)
        n579 = property on="Script" class="MCListbox (strict)"("Value"=w943) -> ()  [unwired: 2 in, 2 out]
        n580 = Not(x=w945) -> (.not. x?=w944:bool)
        n581 = event-data("Discard?"=w944) -> ()  [unwired: 1 in, 1 out]
      }
      event "Script": Shortcut Menu Selection (User) {
        n582 = event-data() -> ("CtlRef"=w955:refnum<vi>, "ItemTag"=w956:string)  [unwired: 1 in, 3 out]
        n583 = property class="MCListbox (strict)"(reference=w955) -> ("Value"=w953:i32)  [unwired: 1 in, 2 out]
        n584 = Unbundle By Name(w951) -> ("state"=w952:refnum<user-event>, "Script"=w954:T16[])
        n585 = case shown="\"Delete Step\"" w956 {
          tunnel: w954 -> [_ w959 w970 w978]
          tunnel: w953 -> [_ w962 w969 w977]
          tunnel: w952 -> [_ w967 w975 w983]
          tunnel: w951 -> [w957 w965 w973 w981]
          tunnel: [w957 w963 w972 w980] -> w950
          frame "False", Default {
          }
          frame "Delete Step" {
            n586 = Delete From Array(array=w959, index=w962) -> (array with subset deleted=w964:T16[])  [unwired: 1 in, 1 out]
            n587 = Array Size(array=w959) -> (size(s)=w960:i32)
            n588 = In Range and Coerce(upper limit=w960, x=w962, lower limit=0) -> (coerced(x)=w958:i32)  [unwired: 1 out]
            n589 = Bundle By Name(cluster=w965, "Script"=w964) -> (w963:T22)
            n590 = property on="Script" class="MCListbox (strict)"("Value"=w958) -> ()  [unwired: 2 in, 2 out]
            n591 = Generate User Event(user event=w967, event data cluster="update script" ("event data")) -> ()  [unwired: 2 in, 2 out]
          }
          frame "Move Down" {
            n592 = Increment(x=w969) -> (x+1=w968:i32)
            n593 = Generate User Event(user event=w975, event data cluster="update script" ("event data")) -> ()  [unwired: 2 in, 2 out]
            n594 = call "CC Swap Script Steps.vi"("index"=w969, "Script in"=w970) -> ("Script out"=w971:T16[])  [unwired: 8 in, 1 out]
            n595 = property on="Script" class="MCListbox (strict)"("Value"=w968) -> ()  [unwired: 2 in, 2 out]
            n596 = Bundle By Name(cluster=w973, "Script"=w971) -> (w972:T22)
          }
          frame "Move Up" {
            n597 = Decrement(x=w977) -> (x-1=w976:i32)
            n598 = Generate User Event(user event=w983, event data cluster="update script" ("event data")) -> ()  [unwired: 2 in, 2 out]
            n599 = call "CC Swap Script Steps.vi"("index"=w976, "Script in"=w978) -> ("Script out"=w979:T16[])  [unwired: 8 in, 1 out]
            n600 = property on="Script" class="MCListbox (strict)"("Value"=w976) -> ()  [unwired: 2 in, 2 out]
            n601 = Bundle By Name(cluster=w981, "Script"=w979) -> (w980:T22)
          }
        }
      }
      event "Script": Shortcut Menu Selection? (App) {
        n602 = event-data() -> ()  [unwired: 1 in, 8 out]
        n603 = event-data("Discard?"=FALSE) -> ()  [unwired: 1 in, 1 out]
      }
      event "Close": Value Change {
        n604 = event-data() -> ()  [unwired: 1 in, 1 out]
        n605 = Unbundle By Name(w989) -> ("Settings"=w987:T18)
        n606 = Unbundle By Name(w987) -> ("Script"=→"script name out":string)
        n607 = call "Rd Wr Script Defaults.vi"("Write? (F:Read)"=TRUE, "Script Settings"=w987) -> ()  [unwired: 8 in, 2 out]
      }
    }
  }
